vi "Single Station Execution.vi"() -> ()   [LabVIEW 2015, in "Single Station Execution.lvlib"]
uses:
  Single Station Execution.lvlib
  Types/Log.SelectedChannels.ctl
  Types/Main.StateVariables.ctl
  Types/INI.Settings.ctl
  <vilib>/NI Veristand/Execution/AlarmManager/AlarmManagerAPI.ctl
  <vilib>/NI Veristand/Execution/DataLogging/IDataLogging Ref.ctl
  <vilib>/NI Veristand/Execution/DataLogging/DataLoggingSpecification Ref.ctl
  Types/Execute.UserEventRefs.ctl
  <vilib>/NI Veristand/Execution/Workspace/SystemStateRegEventRef.ctl
  <vilib>/NI Veristand/Execution/Workspace/Target State Info.ctl
  <vilib>/NI Veristand/Execution/Workspace/Target State.ctl
  Types/Execution.SequenceState.ctl
  <vilib>/NI Veristand/Execution/Workspace/SystemStateEventRef.ctl
  <vilib>/NI Veristand/Execution/Workspace/WorkspaceAPI.ctl
  Types/UDPEngine.QueueCluster.ctl
  Types/UDPEngine.State.ctl
  Types/Results.Value.ctl
  NationalInstruments.VeriStand.RealTimeSequenceDefinitionApi
  <vilib>/NI/AMC/Read Termination Message.vi
  <vilib>/NI/AMC/Update Message Routing Info.vi
  <vilib>/NI/AMC/Create Multiple Messages.vi
  <vilib>/NI/AMC/Create Single Message.vi
  <vilib>/NI/AMC/Globals.vi
  <vilib>/NI/AMC/Send Message.vi
  SubVIs/Main.Constants.vi
  <vilib>/NI Veristand/Execution/Workspace/NI VeriStand - Set Single Channel Value.vi
  <vilib>/NI Veristand/Execution/Workspace/NI_VS Workspace ExecutionAPI.lvlib
  NationalInstruments.VeriStand.ClientAPI
  <vilib>/NI Veristand/Execution/DataLogging/NI_VS Data Logging API.lvlib
  <vilib>/NI/AMC/AMC.lvlib
  <vilib>/NI Veristand/Execution/AlarmManager/NI_VS AlarmManager ExecutionAPI.lvlib
panel:
  in  "ClientPort":u16
  in  "Enable Logging":bool=TRUE
  in  "Log Channels":T1=enum."Aliases"
  in  "Multihead":bool
  out "Status":string
  in  "Station.ID":string="Station_1"
  out "Station ID":string="Station 1"
  in  "NIVS.Gateway IP Address":string="localhost"
  in  "NIVS.Workspace Event":refnum<event-registration>
  in  "ToolTab":enum32{"Enable", "Disable"}(tab)
  in  "Back":bool
  in  "Next":bool
  in  "Pages":enum32{"Metadata", "Alarms", "Execution"}(tab)
  in  "Description":string
  in  "Operator Name":string
  in  "Work Order Number":string
  in  "Cyclic Frequency":dbl
  in  "Number of Cycles":u32
  out "Waveform Preview":waveform(dbl)[](graph)
  in  "Waveform Definition":path
  in  "Revert":bool
  in  "Apply":bool
  in  "Disable Alarms":bool
  out "Monitored Variable":string
  in  "Delay Time":dbl
  in  "Enable State":u16(ring) items=["Disabled", "Enabled", "Tripped", "Delayed Trip", "Indicate"]
  in  "Low":dbl
  in  "High":dbl
  in  "Alarms":i32(listbox)
  in  "Base File Name":string="Log" caption="Base File Name (timestamp included automatically)"
  out "Table":i32(listbox)
  in  "View":enum16{"Graph", "Table"}(ring)
  out "Chart":waveform(dbl)[](graph)
  out "Profile":string
  in  "Run":bool
  in  "Pause":bool
  in  "Abort":bool
  in  "Start Iteration":u32 min=1 max=50
  in  "Start Step":u32 min=1 max=1
  out "Current Iteration":u32 min=1 max=2
  out "Current Step":u32 min=1 max=5
  out "Total Iterations":u32 min=1 max=2
  in  "Skip":bool
  out "Duration":dbl min=1.0 max=3.0
  in  "Open Alarm":bool
  in  "Open Log Directory":bool
  in  "Open Report":bool
  out "Alarm Log Path":path
  in  "Ack":bool
  out "Result":string
  out "Restart Path":path
  out "Report Path":path
  out "Log Directory":path
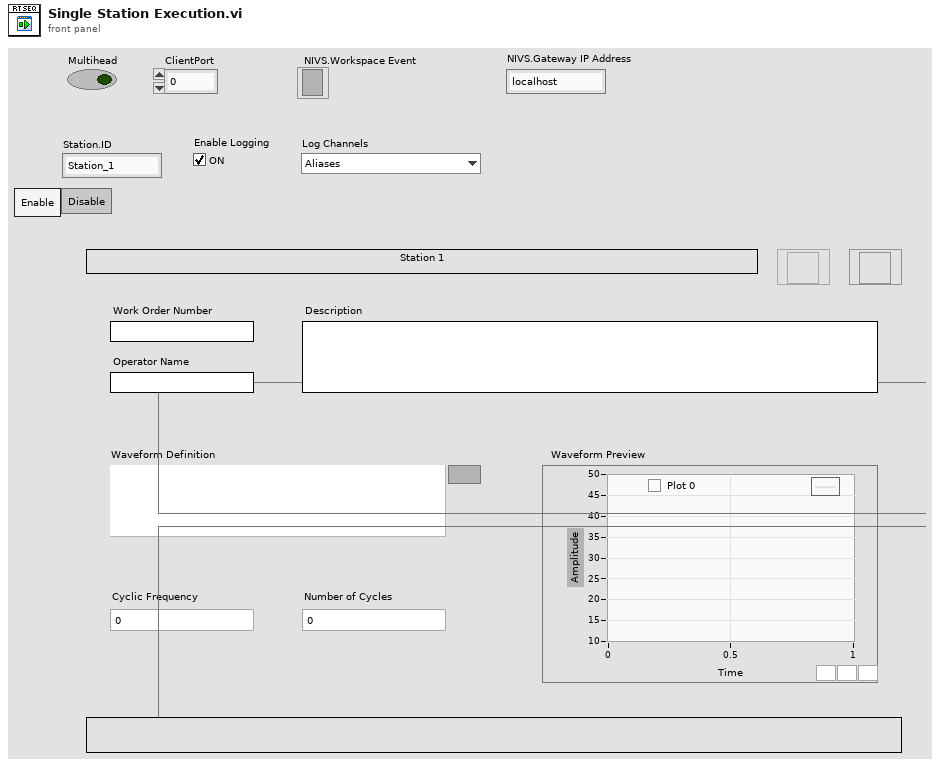
[diagram p1: front panel]
types:
  T1 = typedef "Single Station Execution.lvlib/Log.SelectedChannels.ctl" = enum16{"Channels (No System Channel)", "Aliases", "All"}
  T2 = typedef "Single Station Execution.lvlib/UDPEngine.QueueCluster.ctl" = cluster{"Action":T3, "Channels":string[]}
  T3 = typedef "Single Station Execution.lvlib/UDPEngine.State.ctl" = enum8{"Idle", "Start Acq", "Run", "Stop Acq", "Exit"}
  T4 = typedef "Single Station Execution.lvlib/Execution.SequenceState.ctl" = enum16{"Idle", "Initializing", "Running", "Paused", "Finalizing", "Complete"}
  T5 = typedef "Single Station Execution.lvlib/Main.StateVariables.ctl" = cluster{"Events.State":refnum<user-event>, "Events.Test Result":refnum<user-event>, "Events.Progress":refnum<user-event>, "INI.Settings":T6, "NIVS.AlarmManager":T7, "NIVS.BaseLogPath":path, "NIVS.DataLogManagerRef":T8, "NIVS.DataLogSpecRef":T9, "NIVS.Deployed":bool, "NIVS.Events":T10, "NIVS.GatewayIPAddress":string, "NIVS.DataLogGUID":string, "NIVS.ProfileCallback":refnum<k27>, "NIVS.ProfileRef":refnum<k24>, "NIVS.SequenceState":T4, "NIVS.SystemDefinitionFile":path, "NIVS.SystemStateRefs":T12, "NIVS.WorkspaceManager":T13, "NIVS.EventLogGUID":string, "NIVS.EventLogManagerRef":T8, "NIVS.EventLogSpecRef":T9, "NIVS.BaseToolPath":path, "Restart.Path":path, "Sequence.#ofColumns":i32, "Sequence.Iterations":u32, "Sequence.Channels":string[], "Sequence.ValidConfig?":bool, "Station.ID":string, "UDP.Queue":refnum<queue>, "UI.Abort":refnum<vi>, "UI.Alarms":refnum<vi>, "UI.Apply":refnum<vi>, "UI.Back":refnum<vi>, "UI.BaseFileName":refnum<vi>, "UI.CurrentIteration":refnum<vi>, "UI.CurrentStep":refnum<vi>, "UI.CyclicFrequency":refnum<vi>, "UI.Description":refnum<vi>, "UI.DelayTime":refnum<vi>, "UI.DisableAlarms":refnum<vi>, "UI.Duration":refnum<vi>, "UI.EnableLogging":refnum<vi>, "UI.EnableState":refnum<vi>, "UI.High":refnum<vi>, "UI.LogChannels":refnum<vi>, "UI.Low":refnum<vi>, "UI.MonitoredVariable":refnum<vi>, "UI.Next":refnum<vi>, "UI.NumberOfCycles":refnum<vi>, "UI.OperatorName":refnum<vi>, "UI.Pause":refnum<vi>, "UI.Profile":refnum<vi>, "UI.Revert":refnum<vi>, "UI.Skip":refnum<vi>, "UI.Start":refnum<vi>, "UI.StartIteration":refnum<vi>, "UI.StartStep":refnum<vi>, "UI.TabControl":refnum<vi>, "UI.TotalIterations":refnum<vi>, "UI.WaveformDefinition":refnum<vi>, "UI.WaveformPreview":refnum<vi>, "UI.WorkOrderNumber":refnum<vi>, "UI.Chart":refnum<vi>, "UI.Status":refnum<vi>, "UI.DataView":refnum<vi>, "UI.Table":refnum<vi>, "UI.Multihead":refnum<vi>, "UI.ToolTab":refnum<vi>, "UI.Result":refnum<vi>, "UI.Log Path":refnum<vi>, "UI.ReportPath":refnum<vi>, "UI.RestartPath":refnum<vi>, "UI.AlarmLog":refnum<vi>}
  T6 = typedef "Single Station Execution.lvlib/INI.Settings.ctl" = cluster{"Build Location":path, "LoggingLocation":path, "Sequence.AbortChannel":string, "Sequence.IterationInfoChannel":string, "Sequence.DurationChannel":string, "Sequence.StepInfoChannel":string, "Sequence.SkipChannel":string, "PlotChannels":string[], "Sequence.InitializeScript":path, "Sequence.CleanupScript":path, "Log.DefaultRate":dbl}
  T7 = typedef "NI_VS AlarmManager ExecutionAPI.lvlib/AlarmManagerAPI.ctl" = refnum<k24>
  T8 = typedef "NI_VS Data Logging API.lvlib/IDataLogging Ref.ctl" = refnum<k24>
  T9 = typedef "NI_VS Data Logging API.lvlib/DataLoggingSpecification Ref.ctl" = refnum<k24>
  T10 = typedef "Single Station Execution.lvlib/Execute.UserEventRefs.ctl" = cluster{"SequenceEvent":refnum<event-registration>, "SystemChangeEvent":T11, "WorkspaceEvent":refnum<event-registration>}
  T11 = typedef "NI_VS Workspace ExecutionAPI.lvlib/SystemStateRegEventRef.ctl" = refnum<event-registration>
  T12 = typedef "NI_VS Workspace ExecutionAPI.lvlib/SystemStateEventRef.ctl" = cluster{"CustDatRef":refnum<user-event>, "EvtRef":refnum<k27>, "Target State User Event":refnum<user-event>}
  T13 = typedef "NI_VS Workspace ExecutionAPI.lvlib/WorkspaceAPI.ctl" = refnum<k24>
  T14 = typedef "AMC.lvlib/Message Queue.ctl" = refnum<queue>
  T15 = enum8{"Enabled", "Disabled", "Disabled and Grayed Out"}
  T16 = typedef "Single Station Execution.lvlib/Results.Value.ctl" = enum8{"Passed", "Failed", "Aborted"}
  T17 = typedef "AMC.lvlib/Message.ctl" = cluster{"name":string, "value":string, "attributes":T18, "receiver host":string, "receiver process":string, "source host":string, "source process":string, "priority message":bool, "acknowledge message":bool}
  T18 = typedef "Tools_KeyedArray.lvlib/KeyedArray.ctl" = cluster{"keys":string[], "values":string[]}
  T19 = typedef "NI_VS Workspace ExecutionAPI.lvlib/SystemState.ctl" = u8
  T20 = typedef "Single Station Execution.lvlib/Stimulus.Status.ctl" = cluster{"Restart":bool, "NIVS.SequenceState":T4, "Alarmed?":bool, "Disable?":bool}
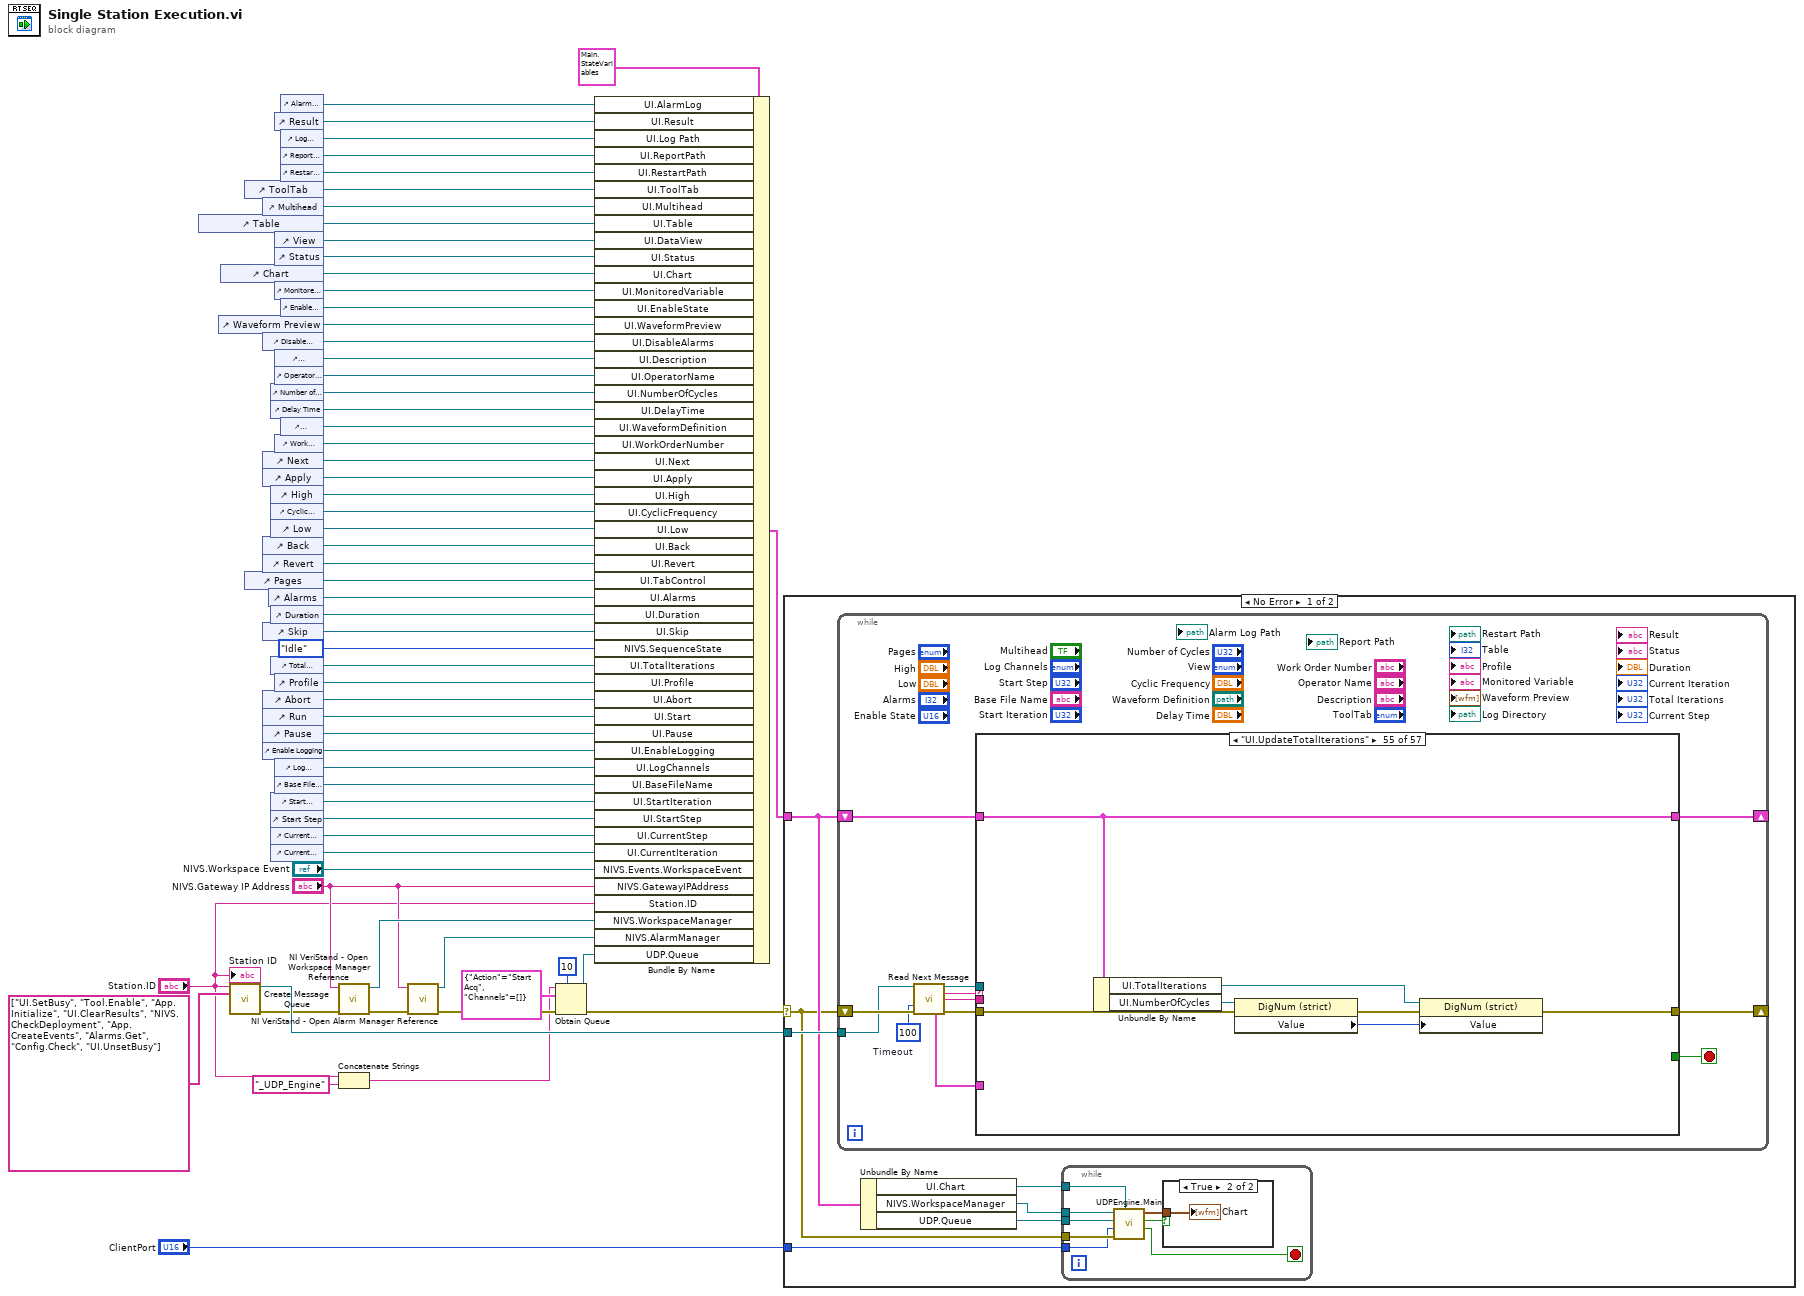
[diagram p0: block diagram]
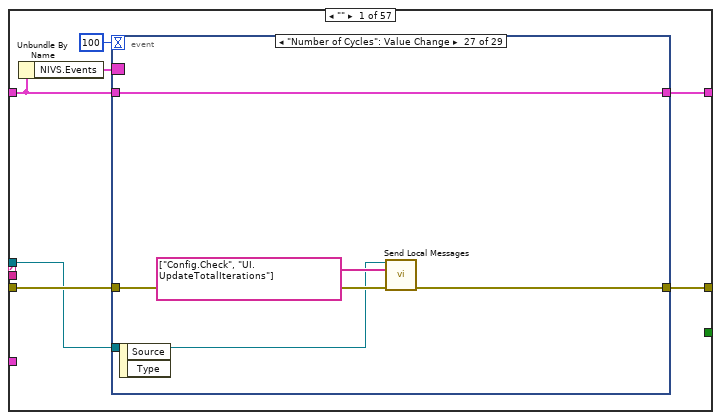
[diagram p3: hidden frame]
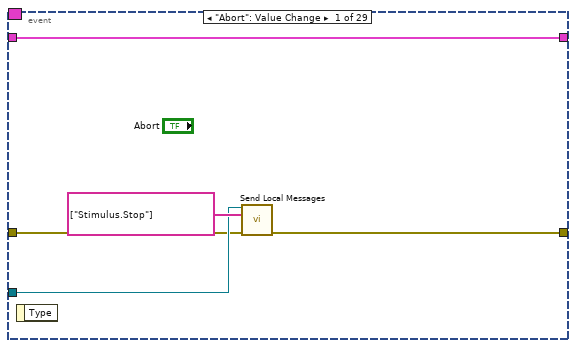
[diagram p4: hidden frame]
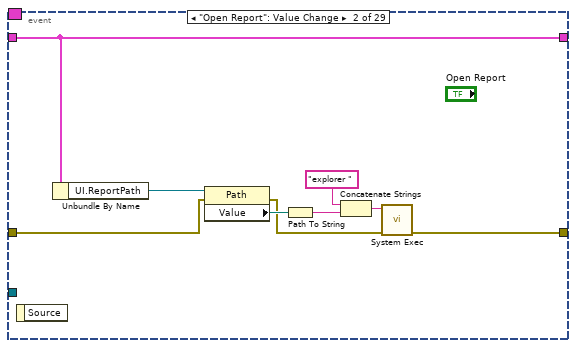
[diagram p5: hidden frame]
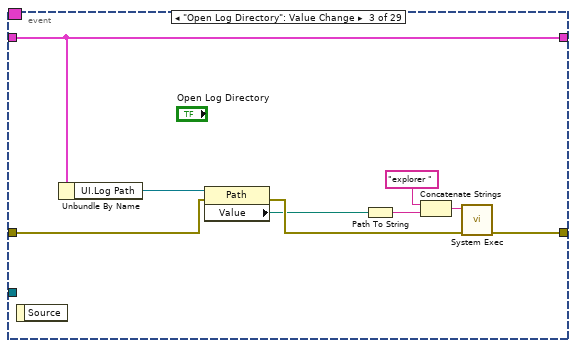
[diagram p6: hidden frame]
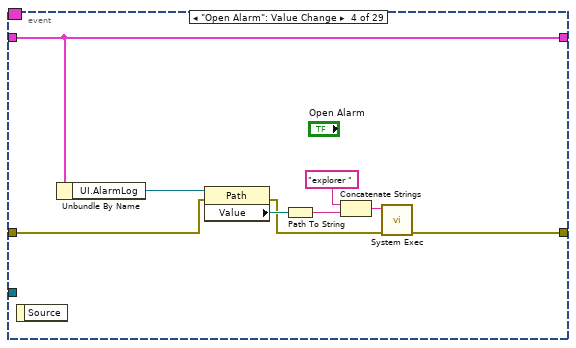
[diagram p7: hidden frame]
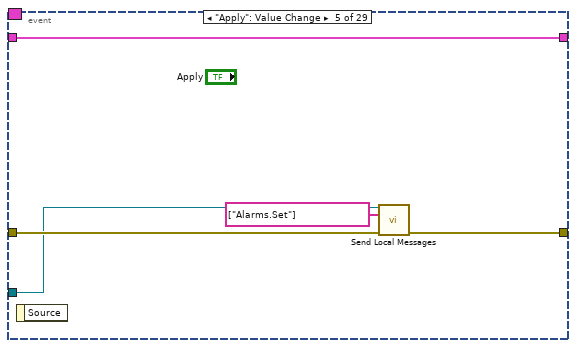
[diagram p8: hidden frame]
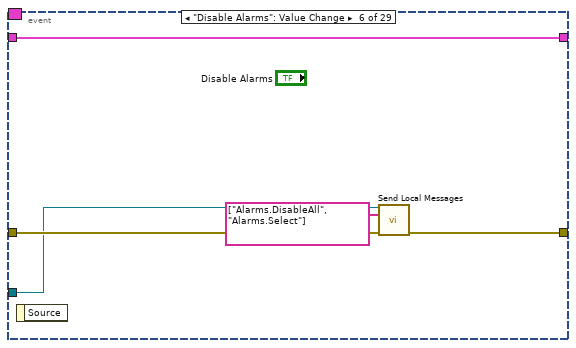
[diagram p9: hidden frame]
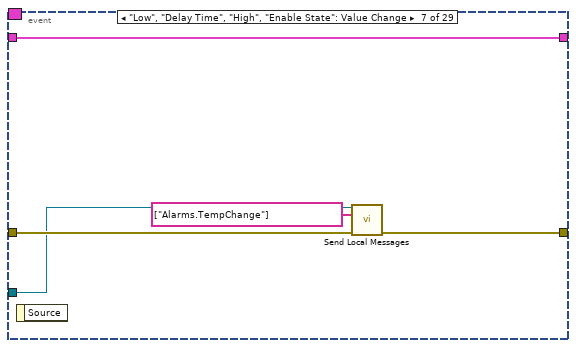
[diagram p10: hidden frame]
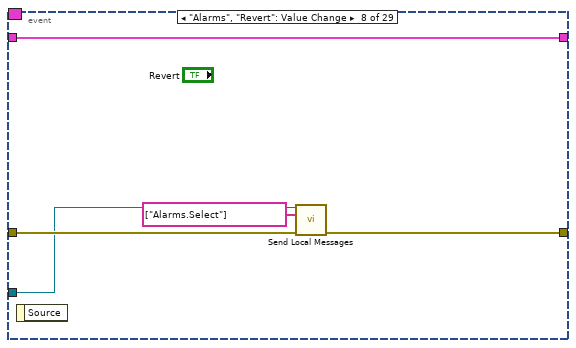
[diagram p11: hidden frame]
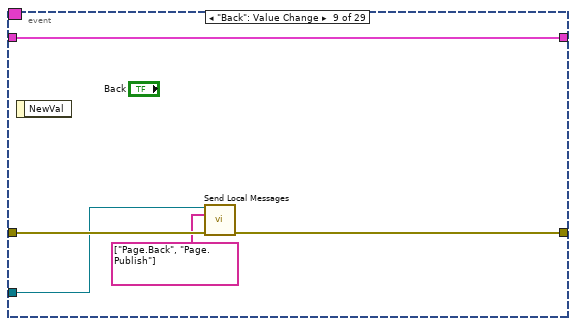
[diagram p12: hidden frame]
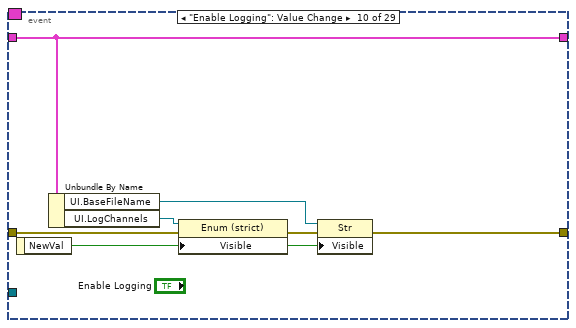
[diagram p13: hidden frame]
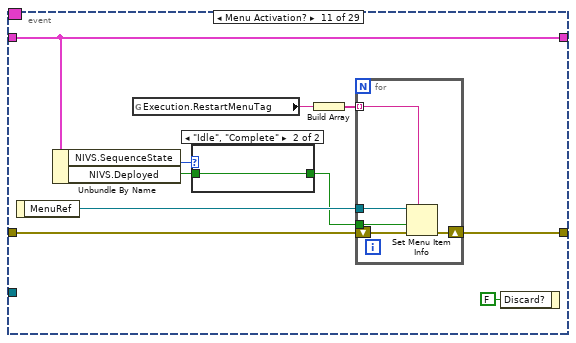
[diagram p14: hidden frame]
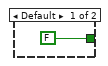
[diagram p15: hidden frame]
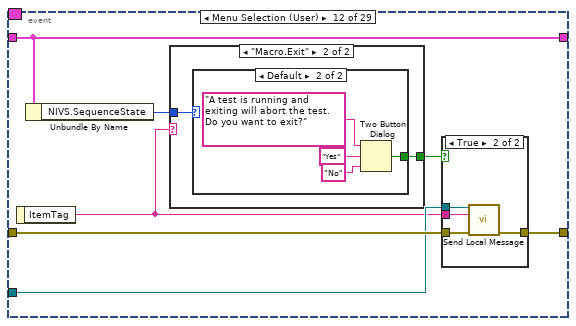
[diagram p16: hidden frame]
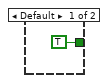
[diagram p18: hidden frame]
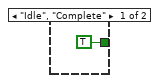
[diagram p19: hidden frame]
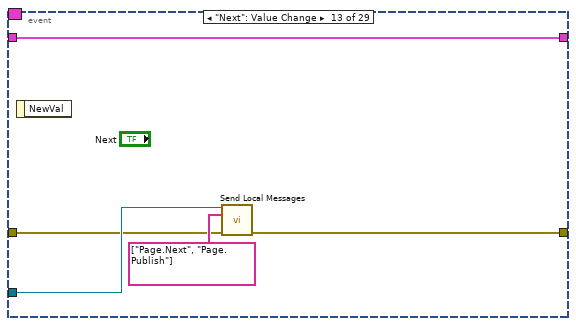
[diagram p20: hidden frame]
diagram:
  n1 = control-ref of="Table"() -> (w12:refnum<vi>)
  n2 = control-ref of="Waveform Preview"() -> (w22:refnum<vi>)
  n3 = control-ref of="Chart"() -> (w14:refnum<vi>)
  n4 = call <vilib>:"Create Message Queue.vi"("message queue name"="Station.ID", "initial message names"=string[] ["UI.SetBusy", "Tool.Enable", "App.Initialize", "UI.ClearResults", "NIVS.CheckDeployment", "App.CreateEvents", "Alarms.Get", "Config.Check", "UI.UnsetBusy"]) -> ("message queue out"=w45:T14, "error out"=w27:errorcluster)  [unwired: 12 in]
  n5 = control-ref of="ToolTab"() -> (w7:refnum<vi>)
  n6 = control-ref of="Pages"() -> (w23:refnum<vi>)
  n7 = control-ref of="Multihead"() -> (w8:refnum<vi>)
  n8 = control-ref of="Disable Alarms"() -> (w30:refnum<vi>)
  n9 = control-ref of="Next"() -> (w36:refnum<vi>)
  n10 = control-ref of="Apply"() -> (w37:refnum<vi>)
  n11 = control-ref of="Back"() -> (w41:refnum<vi>)
  n12 = control-ref of="Revert"() -> (w42:refnum<vi>)
  n13 = control-ref of="Skip"() -> (w47:refnum<vi>)
  n14 = control-ref of="Abort"() -> (w64:refnum<vi>)
  n15 = control-ref of="Run"() -> (w63:refnum<vi>)
  n16 = control-ref of="Pause"() -> (w62:refnum<vi>)
  n17 = control-ref of="Enable Logging"() -> (w61:refnum<vi>)
  n18 = control-ref of="Alarms"() -> (w43:refnum<vi>)
  n19 = control-ref of="Number of Cycles"() -> (w21:refnum<vi>)
  n20 = control-ref of="Delay Time"() -> (w33:refnum<vi>)
  n21 = control-ref of="High"() -> (w38:refnum<vi>)
  n22 = control-ref of="Cyclic Frequency"() -> (w39:refnum<vi>)
  n23 = control-ref of="Low"() -> (w40:refnum<vi>)
  n24 = control-ref of="Duration"() -> (w46:refnum<vi>)
  n25 = control-ref of="Total Iterations"() -> (w50:refnum<vi>)
  n26 = control-ref of="Start Iteration"() -> (w59:refnum<vi>)
  n27 = control-ref of="Start Step"() -> (w58:refnum<vi>)
  n28 = control-ref of="Current Step"() -> (w52:refnum<vi>)
  n29 = control-ref of="Current Iteration"() -> (w51:refnum<vi>)
  n30 = control-ref of="Result"() -> (w3:refnum<vi>)
  n31 = control-ref of="View"() -> (w13:refnum<vi>)
  n32 = control-ref of="Status"() -> (w20:refnum<vi>)
  n33 = control-ref of="Monitored Variable"() -> (w24:refnum<vi>)
  n34 = control-ref of="Description"() -> (w31:refnum<vi>)
  n35 = control-ref of="Operator Name"() -> (w32:refnum<vi>)
  n36 = control-ref of="Work Order Number"() -> (w35:refnum<vi>)
  n37 = control-ref of="Profile"() -> (w56:refnum<vi>)
  n38 = control-ref of="Log Channels"() -> (w60:refnum<vi>)
  n39 = control-ref of="Base File Name"() -> (w49:refnum<vi>)
  n40 = control-ref of="Alarm Log Path"() -> (w2:refnum<vi>)
  n41 = control-ref of="Log Directory"() -> (w4:refnum<vi>)
  n42 = control-ref of="Report Path"() -> (w5:refnum<vi>)
  n43 = control-ref of="Restart Path"() -> (w6:refnum<vi>)
  n44 = control-ref of="Enable State"() -> (w29:refnum<vi>)
  n45 = control-ref of="Waveform Definition"() -> (w34:refnum<vi>)
  n46 = call <vilib>:"NI VeriStand - Open Workspace Manager Reference.vi"("error in (no error)"=w27, "Gateway IP Address (\"\": localhost)"="NIVS.Gateway IP Address") -> ("error out"=w26:errorcluster, "WorkspaceManager"=w53:T13)  [unwired: 8 in]
  n47 = Concatenate Strings("Station.ID", "_UDP_Engine" ("string")) -> (w9:string)
  n48 = call <vilib>:"NI VeriStand - Open Alarm Manager Reference.vi"("error in (no error)"=w26, "Gateway IP Address (\"\": localhost)"="NIVS.Gateway IP Address") -> ("error out"=w17:errorcluster, "AlarmManager"=w28:T7)  [unwired: 8 in]
  n49 = Obtain Queue(max queue size (-1, unlimited)=10, name (unnamed)=w9, element data type=T2 {"Action"=enum."Start Acq", "Channels"=[]}, error in (no error)=w17) -> (queue out=w15:refnum<queue>, error out=w16:errorcluster)  [unwired: 1 in, 1 out]
  n50 = Bundle By Name(cluster=T5 {"Events.State"=refnum, "Events.Test Result"=refnum, "Events.Progress"=refnum, "INI.Settings"={"Build Location"=path "", "LoggingLocation"=path "", "Sequence.AbortChannel"="", "Sequence.IterationInfoChannel"="", "Sequence.DurationChannel"="", "Sequence.StepInfoChannel"="", "Sequence.SkipChannel"="", "PlotChannels"=[], "Sequence.InitializeScript"=path "C:/Simple Sequence Editor/SequenceRepo", "Sequence.CleanupScript"=path "", "Log.DefaultRate"=0.0}, "NIVS.AlarmManager"=refnum, "NIVS.BaseLogPath"=path "", "NIVS.DataLogManagerRef"=refnum, "NIVS.DataLogSpecRef"=refnum, "NIVS.Deployed"=FALSE, "NIVS.Events"={"SequenceEvent"=refnum, "SystemChangeEvent"=refnum, "WorkspaceEvent"=refnum}, "NIVS.GatewayIPAddress"="", "NIVS.DataLogGUID"="", "NIVS.ProfileCallback"=refnum, "NIVS.ProfileRef"=refnum, "NIVS.SequenceState"=enum."Idle", "NIVS.SystemDefinitionFile"=path "", "NIVS.SystemStateRefs"={"CustDatRef"=refnum, "EvtRef"=refnum, "Target State User Event"=refnum}, "NIVS.WorkspaceManager"=refnum, "NIVS.EventLogGUID"="", "NIVS.EventLogManagerRef"=refnum, "NIVS.EventLogSpecRef"=refnum, "NIVS.BaseToolPath"=path "", "Restart.Path"=path "", "Sequence.#ofColumns"=0, "Sequence.Iterations"=0, "Sequence.Channels"=[], "Sequence.ValidConfig?"=FALSE, "Station.ID"="", "UDP.Queue"=refnum, "UI.Abort"=refnum, "UI.Alarms"=refnum, "UI.Apply"=refnum, "UI.Back"=refnum, "UI.BaseFileName"=refnum, "UI.CurrentIteration"=refnum, "UI.CurrentStep"=refnum, "UI.CyclicFrequency"=refnum, "UI.Description"=refnum, "UI.DelayTime"=refnum, "UI.DisableAlarms"=refnum, "UI.Duration"=refnum, "UI.EnableLogging"=refnum, "UI.EnableState"=refnum, "UI.High"=refnum, "UI.LogChannels"=refnum, "UI.Low"=refnum, "UI.MonitoredVariable"=refnum, "UI.Next"=refnum, "UI.NumberOfCycles"=refnum, "UI.OperatorName"=refnum, "UI.Pause"=refnum, "UI.Profile"=refnum, "UI.Revert"=refnum, "UI.Skip"=refnum, "UI.Start"=refnum, "UI.StartIteration"=refnum, "UI.StartStep"=refnum, "UI.TabControl"=refnum, "UI.TotalIterations"=refnum, "UI.WaveformDefinition"=refnum, "UI.WaveformPreview"=refnum, "UI.WorkOrderNumber"=refnum, "UI.Chart"=refnum, "UI.Status"=refnum, "UI.DataView"=refnum, "UI.Table"=refnum, "UI.Multihead"=refnum, "UI.ToolTab"=refnum, "UI.Result"=refnum, "UI.Log Path"=refnum, "UI.ReportPath"=refnum, "UI.RestartPath"=refnum, "UI.AlarmLog"=refnum} ("Cluster"), "UI.AlarmLog"=w2, "UI.Result"=w3, "UI.Log Path"=w4, "UI.ReportPath"=w5, "UI.RestartPath"=w6, "UI.ToolTab"=w7, "UI.Multihead"=w8, "UI.Table"=w12, "UI.DataView"=w13, "UI.Status"=w20, "UI.Chart"=w14, "UI.MonitoredVariable"=w24, "UI.EnableState"=w29, "UI.WaveformPreview"=w22, "UI.DisableAlarms"=w30, "UI.Description"=w31, "UI.OperatorName"=w32, "UI.NumberOfCycles"=w21, "UI.DelayTime"=w33, "UI.WaveformDefinition"=w34, "UI.WorkOrderNumber"=w35, "UI.Next"=w36, "UI.Apply"=w37, "UI.High"=w38, "UI.CyclicFrequency"=w39, "UI.Low"=w40, "UI.Back"=w41, "UI.Revert"=w42, "UI.TabControl"=w23, "UI.Alarms"=w43, "UI.Duration"=w46, "UI.Skip"=w47, "NIVS.SequenceState"=Execution.SequenceState."Idle", "UI.TotalIterations"=w50, "UI.Profile"=w56, "UI.Abort"=w64, "UI.Start"=w63, "UI.Pause"=w62, "UI.EnableLogging"=w61, "UI.LogChannels"=w60, "UI.BaseFileName"=w49, "UI.StartIteration"=w59, "UI.StartStep"=w58, "UI.CurrentStep"=w52, "UI.CurrentIteration"=w51, "NIVS.Events.WorkspaceEvent"="NIVS.Workspace Event", "NIVS.GatewayIPAddress"="NIVS.Gateway IP Address", "Station.ID"="Station.ID", "NIVS.WorkspaceManager"=w53, "NIVS.AlarmManager"=w28, "UDP.Queue"=w15) -> (w57:T5)
  n51 = case shown="No Error" w16 {
    selector: w16 -> [w66 _]
    tunnel: w57 -> [w70 _]
    tunnel: w45 -> [w71 _]
    tunnel: "ClientPort" -> [w65 _]
    frame No Error {
      n52 = while {
        shift-right: [w91] -> _
        shift-left: w70 -> [w92]
        shift-right: [w81] -> _
        shift-left: w66 -> [w90]
        tunnel: w71 -> [w88]
        stop <- w89 stop-if-true
        w87 = 100  # Timeout
        n53 = call <vilib>:"Read Next Message.vi"("message queue in"=w88, "timeout (1 ms)"=w87, "error in"=w90) -> ("message queue out"=w85:T14, "message name"=w84:string, "message value"=w83:string, "message"=w82:T17, "error out"=w86:errorcluster)  [unwired: 5 in, 3 out]
        n54 = case shown="\"UI.UpdateTotalIterations\"" w84 {
          selector: w84 -> [_ _ _ _ _ _ _ _ _ _ _ _ _ _ _ _ _ _ _ _ _ _ _ _ _ _ _ _ _ _ _ _ _ _ _ _ _ w707 _ _ _ _ _ _ _ w775 _ _ _ w790 _ _ _ _ _ _ _]
          tunnel: w92 -> [w95 w361 w373 w378 w383 w386 w393 w398 w401 w405 w416 w429 w440 w449 w459 w465 w492 w505 w525 w544 w569 w574 w588 w593 w598 w606 w609 w630 w661 w665 w670 w675 w676 w682 w687 w693 w699 w709 w715 w722 w730 w741 w747 w768 w774 w779 w780 w783 w786 w793 w807 w817 w827 w855 w866 w874 w876]
          tunnel: [w99 w361 w373 w378 w383 w386 w393 w398 w401 w404 w418 w429 w440 w452 w459 w472 w491 w505 w525 w544 w569 w574 w588 w593 w598 w605 w609 w630 w661 w665 w670 w675 w676 w680 w686 w693 w698 w709 w714 w722 w731 w740 w747 w768 w774 w779 w780 w783 w786 w793 w807 w817 w827 w855 w866 w874 w876] -> w91
          tunnel: [w96 w358 w370 w375 w379 w387 w389 w396 w402 w412 w419 w427 w441 w453 w456 w469 w498 w507 w529 w549 w567 w572 w585 w589 w594 w602 w611 w629 w647 w662 w667 w672 w677 w684 w688 w689 w700 w702 w716 w718 w737 w739 w748 w769 w772 w776 w781 w784 w787 w789 w798 w816 w823 w848 w860 w869 w875] -> w81
          tunnel: w86 -> [w97 w359 w371 w376 w384 w385 w392 w397 w403 w412 w417 w426 w442 w454 w457 w470 w500 w510 w532 w548 w568 w573 w586 w590 w595 w604 w610 w628 w647 w663 w668 w673 w678 w685 w688 w690 w701 w704 w717 w719 w738 w742 w749 w769 w773 w776 w782 w785 w788 w789 w797 w815 w820 w850 w861 w870 w875]
          tunnel: [_ _ _ _ _ _ _ _ _ _ _ _ TRUE _ _ _ _ _ _ _ _ _ _ _ _ _ _ _ _ _ _ _ _ _ _ _ _ _ _ _ _ _ _ _ _ _ _ _ _ _ _ _ _ _ _ _ _] -> w89
          tunnel: w85 -> [w93 _ _ _ w381 _ w388 _ _ _ _ _ w443 _ w458 w460 w497 w504 _ w545 _ w571 w584 w591 w596 w601 _ _ _ _ _ _ _ _ _ _ _ _ _ _ _ _ _ _ _ _ _ _ _ _ _ _ _ _ _ _ _]
          tunnel: w83 -> [_ _ _ _ _ _ _ _ _ _ _ _ _ _ _ _ _ _ _ _ _ _ _ _ _ _ _ _ _ w664 _ _ _ _ _ _ _ _ _ _ _ _ _ _ _ _ _ _ _ _ _ _ w821 _ _ _ _]
          tunnel: w82 -> [_ _ _ _ _ _ _ _ _ _ _ _ _ _ _ _ _ _ _ _ _ _ _ _ _ _ _ _ _ _ _ _ _ _ _ _ _ w713 _ _ _ _ _ _ _ _ _ _ _ _ _ _ _ _ _ _ _]
          frame "" {
            n55 = Unbundle By Name(w95) -> ("NIVS.Events"=w94:T10)
            n56 = event shown="[26] \"Number of Cycles\": Value Change" {
              selector: w94 -> [_ _ _ _ _ _ _ _ _ _ _ _ _ _ _ _ _ _ _ _ _ _ _ _ _ _ _ _ _]
              dyn-events: _ -> [_ _ _ _ _ _ _ _ _ _ _ _ _ _ _ _ _ _ _ _ _ _ _ _ _ _ _ _ _]
              timeout: 100 -> [_ _ _ _ _ _ _ _ _ _ _ _ _ _ _ _ _ _ _ _ _ _ _ _ _ _ _ _ _]
              tunnel: [w104 w113 w122 w131 w136 w141 w146 w151 w156 w163 w173 w181 w205 w211 w217 w225 w244 w245 w263 w269 w279 w302 w306 w313 w318 w323 w328 w337 w345] -> w99
              tunnel: w95 -> [w104 w113 w122 w131 w136 w141 w146 w151 w156 w163 w173 w181 w205 w211 w217 w225 w244 w256 w263 w270 w279 w302 w306 w313 w318 w323 w328 w337 w345]
              tunnel: [w100 w105 w115 w123 w133 w138 w144 w149 w154 w157 w169 w186 w203 w208 w215 w218 w243 w250 w261 w264 w275 w297 w307 w311 w316 w320 w325 w332 w342] -> w96
              tunnel: w97 -> [w101 w111 w120 w129 w134 w139 w145 w150 w155 w161 w170 w187 w201 w209 w216 w222 w243 w246 w262 w268 w276 w298 w308 w312 w317 w321 w326 w333 w343]
              tunnel: w93 -> [w102 _ _ _ w132 w137 w143 w148 w153 _ _ w185 w202 w207 w214 w220 _ w248 w260 w267 _ w299 _ w309 w314 w319 w324 _ w341]
              event "Abort": Value Change {
                n57 = event-data() -> ()  [unwired: 1 in, 1 out]
                n58 = call <vilib>:"Send Local Messages.vi"("message queue in"=w102, "message names"=string[] ["Stimulus.Stop"] ("array"), "error in"=w101) -> ("error out"=w100:errorcluster)  [unwired: 10 in, 2 out]
              }
              event "Open Report": Value Change {
                n59 = event-data() -> ()  [unwired: 1 in, 1 out]
                n60 = Unbundle By Name(w113) -> ("UI.ReportPath"=w112:refnum<vi>)
                n61 = property class="Path"(reference=w112, error in=w111) -> (error out=w106:errorcluster, "Value"=w107:path)  [unwired: 1 out]
                n62 = Path To String(path=w107) -> (string=w110:string)
                n63 = Concatenate Strings("explorer " ("string"), w110) -> (w108:string)
                n64 = call <vilib>:"System Exec.vi"("error in (no error)"=w106, "command line"=w108) -> ("error out"=w105:errorcluster)  [unwired: 6 in, 3 out]
              }
              event "Open Log Directory": Value Change {
                n65 = event-data() -> ()  [unwired: 1 in, 1 out]
                n66 = Unbundle By Name(w122) -> ("UI.Log Path"=w121:refnum<vi>)
                n67 = property class="Path"(reference=w121, error in=w120) -> (error out=w116:errorcluster, "Value"=w114:path)  [unwired: 1 out]
                n68 = Path To String(path=w114) -> (string=w119:string)
                n69 = Concatenate Strings("explorer " ("string"), w119) -> (w117:string)
                n70 = call <vilib>:"System Exec.vi"("error in (no error)"=w116, "command line"=w117) -> ("error out"=w115:errorcluster)  [unwired: 6 in, 3 out]
              }
              event "Open Alarm": Value Change {
                n71 = event-data() -> ()  [unwired: 1 in, 1 out]
                n72 = Unbundle By Name(w131) -> ("UI.AlarmLog"=w130:refnum<vi>)
                n73 = property class="Path"(reference=w130, error in=w129) -> (error out=w124:errorcluster, "Value"=w125:path)  [unwired: 1 out]
                n74 = Path To String(path=w125) -> (string=w128:string)
                n75 = Concatenate Strings("explorer " ("string"), w128) -> (w126:string)
                n76 = call <vilib>:"System Exec.vi"("error in (no error)"=w124, "command line"=w126) -> ("error out"=w123:errorcluster)  [unwired: 6 in, 3 out]
              }
              event "Apply": Value Change {
                n77 = event-data() -> ()  [unwired: 1 in, 1 out]
                n78 = call <vilib>:"Send Local Messages.vi"("message queue in"=w132, "message names"=string[] ["Alarms.Set"], "error in"=w134) -> ("error out"=w133:errorcluster)  [unwired: 10 in, 2 out]
              }
              event "Disable Alarms": Value Change {
                n79 = event-data() -> ()  [unwired: 1 in, 1 out]
                n80 = call <vilib>:"Send Local Messages.vi"("message queue in"=w137, "message names"=string[] ["Alarms.DisableAll", "Alarms.Select"], "error in"=w139) -> ("error out"=w138:errorcluster)  [unwired: 10 in, 2 out]
              }
              event "Low", "Delay Time", "High", "Enable State": Value Change {
                n81 = event-data() -> ()  [unwired: 1 in, 1 out]
                n82 = call <vilib>:"Send Local Messages.vi"("message queue in"=w143, "message names"=string[] ["Alarms.TempChange"], "error in"=w145) -> ("error out"=w144:errorcluster)  [unwired: 10 in, 2 out]
              }
              event "Alarms", "Revert": Value Change {
                n83 = event-data() -> ()  [unwired: 1 in, 1 out]
                n84 = call <vilib>:"Send Local Messages.vi"("message queue in"=w148, "message names"=string[] ["Alarms.Select"], "error in"=w150) -> ("error out"=w149:errorcluster)  [unwired: 10 in, 2 out]
              }
              event "Back": Value Change {
                n85 = event-data() -> ()  [unwired: 1 in, 1 out]
                n86 = call <vilib>:"Send Local Messages.vi"("message queue in"=w153, "message names"=string[] ["Page.Back", "Page.Publish"], "error in"=w155) -> ("error out"=w154:errorcluster)  [unwired: 10 in, 2 out]
              }
              event "Enable Logging": Value Change {
                n87 = event-data() -> ("NewVal"=w158:bool)  [unwired: 1 in]
                n88 = Unbundle By Name(w163) -> ("UI.BaseFileName"=w159:refnum<vi>, "UI.LogChannels"=w162:refnum<vi>)
                n89 = property class="Enum (strict)"(reference=w162, error in=w161, "Visible"=w158) -> (error out=w160:errorcluster)  [unwired: 1 out]
                n90 = property class="Str"(reference=w159, error in=w160, "Visible"=w158) -> (error out=w157:errorcluster)  [unwired: 1 out]
              }
              event Menu Activation? {
                n91 = event-data() -> ("MenuRef"=w171:refnum<k9>)  [unwired: 1 in]
                n92 = Unbundle By Name(w173) -> ("NIVS.SequenceState"=w172:T4, "NIVS.Deployed"=w164:bool)
                n93 = global read "Main.Constants.vi" "Execution.RestartMenuTag"() -> (w167:string)
                n94 = case shown="\"Idle\", \"Complete\"" w172 {
                  tunnel: [FALSE w180] -> w168
                  tunnel: w164 -> [_ w180]
                  frame Default {
                  }
                  frame "Idle", "Complete" {
                  }
                }
                n95 = Build Array(w167) -> (w166:string[])
                n96 = for {
                  tunnel: w171 -> [w178]
                  shift-right: [w176] -> w169
                  shift-left: w170 -> [w177]
                  tunnel: w168 -> [w175]
                  tunnel: w166 -> [w174] mode=indexing
                  n97 = Set Menu Item Info(7:w174, 8:w177, 9:w175, 11:w178) -> (0:w176:errorcluster)  [unwired: 3 in, 1 out]
                }
                n98 = event-data("Discard?"=FALSE) -> ()  [unwired: 1 in, 1 out]
              }
              event Menu Selection (User) {
                n99 = event-data() -> ("ItemTag"=w184:string)  [unwired: 1 in]
                n100 = Unbundle By Name(w181) -> ("NIVS.SequenceState"=w182:T4)
                n101 = case shown="\"Macro.Exit\"" w184 {
                  tunnel: [TRUE ("T button?") w195] -> w183
                  tunnel: w182 -> [_ w194]
                  frame Default {
                  }
                  frame "Macro.Exit" {
                    n102 = case shown="Default" w194 {
                      tunnel: [TRUE ("T button?") w197] -> w195
                      frame "Idle", "Complete" {
                      }
                      frame Default {
                        n103 = Two Button Dialog(message="A test is running and exiting will abort the test. Do you want to exit?", 1:"No" ("F button name (\"Cancel\")"), 2:"Yes" ("T button name (\"OK\")")) -> (T button?=w197:bool)
                      }
                    }
                  }
                }
                n104 = case shown="True" w183 {
                  tunnel: w187 -> [w188 w192]
                  tunnel: [w188 w191] -> w186
                  tunnel: w185 -> [_ w190]
                  tunnel: w184 -> [_ w189]
                  frame False {
                  }
                  frame True {
                    n105 = call <vilib>:"Send Local Message.vi"("message queue in"=w190, "message name"=w189, "error in"=w192) -> ("error out"=w191:errorcluster)  [unwired: 10 in, 2 out]
                  }
                }
              }
              event "Next": Value Change {
                n106 = event-data() -> ()  [unwired: 1 in, 1 out]
                n107 = call <vilib>:"Send Local Messages.vi"("message queue in"=w202, "message names"=string[] ["Page.Next", "Page.Publish"], "error in"=w201) -> ("error out"=w203:errorcluster)  [unwired: 10 in, 2 out]
              }
              event Panel Close? {
                n108 = event-data() -> ()  [unwired: 1 in, 1 out]
                n109 = Build Array("Macro.Exit") -> (w206:string[])
                n110 = call <vilib>:"Send Local Messages.vi"("message queue in"=w207, "message names"=w206, "error in"=w209) -> ("error out"=w208:errorcluster)  [unwired: 10 in, 2 out]
                n111 = event-data("Discard?"=TRUE) -> ()  [unwired: 1 in, 1 out]
              }
              event "Pause": Value Change {
                n112 = event-data() -> ()  [unwired: 1 in, 1 out]
                n113 = call <vilib>:"Send Local Messages.vi"("message queue in"=w214, "message names"=string[] ["Stimulus.Pause"] ("array"), "error in"=w216) -> ("error out"=w215:errorcluster)  [unwired: 10 in, 2 out]
              }
              event "Run": Value Change {
                n114 = event-data() -> ("CtlRef"=w223:refnum<vi>)  [unwired: 1 in]
                n115 = Unbundle By Name(w225) -> ("NIVS.SequenceState"=w224:T4)
                n116 = property class="Bool"(reference=w223, error in=w222) -> (error out=w219:errorcluster, "BoolText.Text"=w221:string)  [unwired: 1 out]
                n117 = case shown="\"Run\", Default" w221 {
                  tunnel: w224 -> [_ w233]
                  tunnel: w220 -> [w228 w232]
                  tunnel: w219 -> [w227 w231]
                  tunnel: [w226 w230] -> w218
                  frame "Restart" {
                    n118 = call <vilib>:"Send Local Messages.vi"("message queue in"=w228, "message names"=string[] ["Macro.Restart"], "error in"=w227) -> ("error out"=w226:errorcluster)  [unwired: 10 in, 2 out]
                  }
                  frame "Run", Default {
                    n119 = case shown="\"Idle\"" w233 {
                      tunnel: w232 -> [w236 _ w241]
                      tunnel: w231 -> [w235 w238 w242]
                      tunnel: [w234 w238 w240] -> w230
                      frame "Paused" {
                        n120 = call <vilib>:"Send Local Messages.vi"("message queue in"=w236, "message names"=string[] ["Stimulus.Continue"] ("array"), "error in"=w235) -> ("error out"=w234:errorcluster)  [unwired: 10 in, 2 out]
                      }
                      frame Default {
                      }
                      frame "Idle" {
                        n121 = call <vilib>:"Send Local Messages.vi"("message queue in"=w241, "message names"=string[] ["Macro.Run"] ("array"), "error in"=w242) -> ("error out"=w240:errorcluster)  [unwired: 10 in, 2 out]
                      }
                    }
                  }
                }
              }
              event User Event {
                n122 = event-data() -> ()  [unwired: 1 in, 1 out]
              }
              event User Event {
                n123 = event-data() -> ("Test Result"=w257:path)  [unwired: 1 in]
                n124 = call "Restart.HandleSequenceFinishedEvent.vi"("error in (no error)"=w246, "results path"=w257, "State Variables"=w256) -> ("error out"=w251:errorcluster, "Restart?"=w255:bool, "State Variables out"=w245:T5)  [unwired: 6 in]
                n125 = Select(t="UI.StimulusRestart", s=w255, f="UI.StimulusComplete") -> (s? t:f=w252:string)
                n126 = Build Array (concatenate)(string[] ["Stimulus.Close", "Stimulus.UnregisterCallbacks", "Acq.Stop"], w252, "Tool.Disable" ("element")) -> (w249:string[])
                n127 = call <vilib>:"Send Local Messages.vi"("message queue in"=w248, "message names"=w249, "error in"=w251) -> ("error out"=w250:errorcluster)  [unwired: 10 in, 2 out]
              }
              event "Ack": Value Change {
                n128 = event-data() -> ()  [unwired: 1 in, 1 out]
                n129 = call <vilib>:"Send Local Messages.vi"("message queue in"=w260, "message names"=string[] ["Tool.Enable", "UI.ClearResults"], "error in"=w262) -> ("error out"=w261:errorcluster)  [unwired: 10 in, 2 out]
              }
              event User Event {
                n130 = event-data() -> ("State"=w265:i32)  [unwired: 1 in]
                n131 = Bundle By Name(cluster=w270, "NIVS.SequenceState"=w265) -> (w269:T5)
                n132 = call <vilib>:"Send Local Messages.vi"("message queue in"=w267, "message names"=string[] ["UI.UpdateState", "UI.UpdateStatus"] ("array"), "error in"=w268) -> ("error out"=w264:errorcluster)  [unwired: 10 in, 2 out]
              }
              event "Skip": Value Change {
                n133 = event-data() -> ()  [unwired: 1 in, 1 out]
                n134 = Unbundle By Name(w279) -> ("Sequence.ValidConfig?"=w273:bool, "NIVS.Deployed"=w272:bool, "NIVS.SequenceState"=w274:T4, "NIVS.WorkspaceManager"=w278:T13, "INI.Settings.Sequence.SkipChannel"=w277:string)
                n135 = Compound Arithmetic op=AND(w273, w272) -> (w271:bool)
                n136 = case shown="True" w271 {
                  tunnel: w278 -> [_ w283]
                  tunnel: w276 -> [w280 w285]
                  tunnel: [w280 w284] -> w275
                  tunnel: w277 -> [_ w282]
                  tunnel: w274 -> [_ w281]
                  frame False {
                  }
                  frame True {
                    n137 = case shown="Default" w281 {
                      tunnel: w285 -> [w286 w290]
                      tunnel: [w286 w289] -> w284
                      tunnel: w283 -> [_ w288]
                      tunnel: w282 -> [_ w287]
                      frame "Idle", "Complete" {
                      }
                      frame Default {
                        n138 = case shown="Default" w287 {
                          selector: w287 -> [_ w292]
                          tunnel: w290 -> [w291 w296]
                          tunnel: [w291 w295] -> w289
                          tunnel: w288 -> [_ w294]
                          frame "" {
                          }
                          frame Default {
                            n139 = call-poly <vilib>:"NI VeriStand - Set Channel Value.vi"("error in (no error)"=w296, "Value"=1.0, "Channel"=w292, "WorkspaceManager in"=w294) -> ("error out"=w295:errorcluster)  [unwired: 6 in, 1 out]
                          }
                        }
                      }
                    }
                  }
                }
              }
              event User Event {
                n140 = event-data() -> ()  [unwired: 1 in, 1 out]
                n141 = Unbundle By Name(w302) -> ("NIVS.SequenceState"=w301:T4)
                n142 = case shown="\"Idle\", \"Complete\"" w301 {
                  tunnel: [string[] ["Stimulus.CacheRestart", "NIVS.CheckDeployment"] w305] -> w300
                  frame Default {
                  }
                  frame "Idle", "Complete" {
                    n143 = Build Array("NIVS.CheckDeployment") -> (w305:string[])
                  }
                }
                n144 = call <vilib>:"Send Local Messages.vi"("message queue in"=w299, "message names"=w300, "error in"=w298) -> ("error out"=w297:errorcluster)  [unwired: 10 in, 2 out]
              }
              event Timeout {
                n145 = event-data() -> ()  [unwired: 1 in, 1 out]
                n146 = call "Stimulus.GetStatusInfo.vi"("error in (no error)"=w308, "Cluster"=w306) -> ("error out"=w307:errorcluster)  [unwired: 9 in]
              }
              event "Waveform Definition": Value Change {
                n147 = event-data() -> ()  [unwired: 1 in, 2 out]
                n148 = call <vilib>:"Send Local Messages.vi"("message queue in"=w309, "message names"=string[] ["Sequence.Open", "UI.UpdatePreview", "Config.Check"], "error in"=w312) -> ("error out"=w311:errorcluster)  [unwired: 10 in, 2 out]
              }
              event "Cyclic Frequency": Value Change {
                n149 = event-data() -> ()  [unwired: 1 in, 2 out]
                n150 = call <vilib>:"Send Local Messages.vi"("message queue in"=w314, "message names"=string[] ["UI.UpdatePreview", "Config.Check"], "error in"=w317) -> ("error out"=w316:errorcluster)  [unwired: 10 in, 2 out]
              }
              event "Operator Name", "Work Order Number", "Description": Value Change {
                n151 = event-data() -> ()  [unwired: 1 in, 2 out]
                n152 = call <vilib>:"Send Local Messages.vi"("message queue in"=w319, "message names"=string[] ["Config.Check"], "error in"=w321) -> ("error out"=w320:errorcluster)  [unwired: 10 in, 2 out]
              }
              event "Number of Cycles": Value Change {
                n153 = event-data() -> ()  [unwired: 1 in, 2 out]
                n154 = call <vilib>:"Send Local Messages.vi"("message queue in"=w324, "message names"=string[] ["Config.Check", "UI.UpdateTotalIterations"], "error in"=w326) -> ("error out"=w325:errorcluster)  [unwired: 10 in, 2 out]
              }
              event "View": Value Change {
                n155 = event-data() -> ("NewVal"=w331:enum16{"Graph", "Table"})  [unwired: 1 in]
                n156 = case shown="\"Graph\"" w331 {
                  tunnel: [TRUE FALSE] -> w330
                  frame "Graph" {
                  }
                  frame "Table" {
                  }
                }
                n157 = Unbundle By Name(w337) -> ("UI.Table"=w335:refnum<vi>, "UI.Chart"=w336:refnum<vi>)
                n158 = property class="WFChart (strict)"(reference=w336, error in=w333, "Visible"=w330) -> (error out=w334:errorcluster)  [unwired: 1 out]
                n159 = Not(x=w330) -> (.not. x?=w329:bool)
                n160 = property class="MCListbox (strict)"(reference=w335, error in=w334, "Visible"=w329) -> (error out=w332:errorcluster)  [unwired: 1 out]
              }
              event User Event {
                n161 = event-data() -> ("Workspace Event"=w340:string)  [unwired: 1 in]
                n162 = Unbundle By Name(w345) -> ("NIVS.SequenceState"=w344:T4)
                n163 = Equal?(x="Shut Down" ("y"), y=w340) -> (x = y?=w346:bool)
                n164 = case shown="True" w346 {
                  tunnel: w344 -> [_ _]
                  tunnel: w343 -> [w348 w353]
                  tunnel: [w348 w352] -> w342
                  tunnel: w341 -> [_ w351]
                  frame False {
                  }
                  frame True {
                    n165 = Build Array("Macro.Exit" ("y")) -> (w350:string[])
                    n166 = call <vilib>:"Send Local Messages.vi"("message queue in"=w351, "message names"=w350, "error in"=w353) -> ("error out"=w352:errorcluster)  [unwired: 10 in, 2 out]
                  }
                }
              }
            }
          }
          frame "Acq.Start" {
            n167 = Unbundle By Name(w361) -> ("UDP.Queue"=w360:refnum<queue>, "Sequence.Channels"=w356:string[], "INI.Settings.PlotChannels"=w357:string[])
            n168 = Build Array (concatenate)(w356, w357) -> (w355:string[])
            n169 = Empty Array?(array=w355) -> (empty?=w354:bool)
            n170 = case shown="False" w354 {
              tunnel: w360 -> [w367 _]
              tunnel: w359 -> [w364 w368]
              tunnel: [w363 w368] -> w358
              tunnel: w355 -> [w362 _]
              frame False {
                n171 = Bundle By Name(cluster=T2 {"Action"=enum."Start Acq", "Channels"=[]} ("element"), "Channels"=w362) -> (w365:T2)
                n172 = Enqueue Element(queue=w367, element=w365, error in (no error)=w364) -> (error out=w363:errorcluster)  [unwired: 1 in, 2 out]
              }
              frame True {
              }
            }
          }
          frame "Acq.Stop" {
            n173 = Unbundle By Name(w373) -> ("UDP.Queue"=w372:refnum<queue>)
            n174 = Enqueue Element(queue=w372, element=T2 {"Action"=enum."Stop Acq", "Channels"=[]}, error in (no error)=w371) -> (error out=w370:errorcluster)  [unwired: 1 in, 2 out]
          }
          frame "Acq.Exit" {
            n175 = Unbundle By Name(w378) -> ("UDP.Queue"=w377:refnum<queue>)
            n176 = Enqueue Element(queue=w377, element=T2 {"Action"=enum."Exit", "Channels"=[]}, error in (no error)=w376) -> (error out=w375:errorcluster)  [unwired: 1 in, 2 out]
          }
          frame "Alarms.Get" {
            n177 = call "Alarms.Get.vi"("error in (no error)"=w384, "Cluster"=w383) -> ("error out"=w380:errorcluster)  [unwired: 9 in]
            n178 = call <vilib>:"Send Local Message.vi"("message queue in"=w381, "message name"="Alarms.Select", "error in"=w380) -> ("error out"=w379:errorcluster)  [unwired: 10 in, 2 out]
          }
          frame "Alarms.Select" {
            n179 = call "Alarms.Select.vi"("error in (no error)"=w385, "Cluster"=w386) -> ("error out"=w387:errorcluster)  [unwired: 9 in]
          }
          frame "Alarms.Set" {
            n180 = call "Alarms.Set.vi"("error in (no error)"=w392, "Cluster"=w393) -> ("error out"=w390:errorcluster)  [unwired: 9 in]
            n181 = call <vilib>:"Send Local Message.vi"("message queue in"=w388, "message name"="Alarms.Select", "error in"=w390) -> ("error out"=w389:errorcluster)  [unwired: 10 in, 2 out]
          }
          frame "Alarms.TempChange" {
            w399 = T15."Enabled" ("Disabled")
            n182 = Unbundle By Name(w398) -> ("UI.Apply"=w395:refnum<vi>, "UI.Revert"=w394:refnum<vi>)
            n183 = property class="Bool"(reference=w394, error in=w397, "DisabledEnum"=w399) -> (error out=w400:errorcluster)  [unwired: 1 out]
            n184 = property class="Bool"(reference=w395, error in=w400, "DisabledEnum"=w399) -> (error out=w396:errorcluster)  [unwired: 1 out]
          }
          frame "Alarms.DisableAll" {
            n185 = call "Alarms.DisableALl.vi"("error in (no error)"=w403, "Cluster"=w401) -> ("error out"=w402:errorcluster)  [unwired: 9 in]
          }
          frame "App.CloseReferences" {
            n186 = flat-sequence {
              tunnel: [w414] -> w404
              tunnel: w405 -> [w414]
              tunnel: [w413] -> _
              frame #0 {
                n187 = invoke class="VI" method="FP.Close"() -> (error out=w413:errorcluster)  [unwired: 3 in, 2 out]
                n188 = Wait (ms)(milliseconds to wait=u32 500) -> ()  [unwired: 1 out]
              }
            }
            n189 = Unbundle By Name(w404) -> ("Events.State"=w409:refnum<user-event>, "Events.Test Result"=w410:refnum<user-event>, "Events.Progress"=w411:refnum<user-event>, "NIVS.Events"=w406:T10, "NIVS.SystemStateRefs"=w408:T12, "NIVS.WorkspaceManager"=w407:T13)
            n190 = call <vilib>:"NI VeriStand - Close Workspace Manager Reference.vi"("WorkspaceManager"=w407) -> ()  [unwired: 10 in, 1 out]
            n191 = call <vilib>:"NI VeriStand - Close Engine State Change Notification.vi"("SystemStateRefs"=w408) -> ()  [unwired: 10 in, 1 out]
            n192 = Unregister For Events(event registration refnum=w406) -> ()  [unwired: 1 in, 1 out]
            n193 = Destroy User Event(user event=w411) -> ()  [unwired: 1 in, 1 out]
            n194 = Destroy User Event(user event=w410) -> ()  [unwired: 1 in, 1 out]
            n195 = Destroy User Event(user event=w409) -> ()  [unwired: 1 in, 1 out]
          }
          frame "App.CreateEvents" {
            n196 = call "Execute.CreateEvents.vi"("error in (no error)"=w417, "Cluster in"=w416) -> ("error out"=w419:errorcluster, "Cluster out"=w418:T5)  [unwired: 8 in]
          }
          frame "App.CreateFolders" {
            n197 = Unbundle By Name(w429) -> ("NIVS.BaseToolPath"=w422:path, "NIVS.BaseLogPath"=w428:path)
            n198 = Build Path(base path=w422, name or relative path="Configurations") -> (appended path=w421:path)
            n199 = flat-sequence {
              tunnel: w428 -> [w433]
              tunnel: w426 -> [w432]
              tunnel: [w432] -> w425
              tunnel: [w431] -> w424
              tunnel: w421 -> [w430]
              tunnel: [w430] -> w420
              tunnel: [w436] -> _
              tunnel: [w437] -> w427
              tunnel: w425 -> [w437]
              tunnel: w424 -> [w436]
              tunnel: w420 -> [w435]
              tunnel: [w434] -> _
              frame #0 {
                n200 = Create Folder(path (use dialog)=w433) -> (error out=w431:errorcluster)  [unwired: 2 in, 2 out]
              }
              frame #1 {
                n201 = Create Folder(path (use dialog)=w435) -> (error out=w434:errorcluster)  [unwired: 2 in, 2 out]
              }
            }
          }
          frame "App.Exit" {
            n202 = call <vilib>:"Destroy Message Queue.vi"("message queue in"=w443, "error in"=w442) -> ("error out"=w441:errorcluster)  [unwired: 11 in, 2 out]
            n203 = Unbundle By Name(w440) -> ("UI.Multihead"=w439:refnum<vi>)
            n204 = property class="Bool (strict)"(reference=w439, "Value"=FALSE) -> ()  [unwired: 1 in, 2 out]
          }
          frame "App.Initialize" {
            n205 = call "Execute.Initialize.vi"("error in (no error)"=w454, "Cluster"=w449) -> ("error out"=w447:errorcluster)  [unwired: 9 in]
            n206 = call "Tool.GetPath.vi"("error in (no error)"=w447, "Cluster"=w449) -> ("error out"=w446:errorcluster, "path"=w445:path)  [unwired: 8 in]
            n207 = call "INI.GetSettings.vi"("error in (no error)"=w446, "INI Folder Location"=w445, "State Variables"=w449) -> ("error out"=w453:errorcluster, "INI.Settings"=w451:T6)  [unwired: 7 in]
            n208 = Bundle By Name(cluster=w449, "NIVS.BaseToolPath"=w445, "Sequence.Channels"=string[] [], "Restart.Path"=path "", "INI.Settings"=w451) -> (w452:T5)
          }
          frame "App.New" {
            n209 = call <vilib>:"Send Local Message.vi"("message queue in"=w458, "message name"="Macro.New", "error in"=w457) -> ("error out"=w456:errorcluster)  [unwired: 10 in, 2 out]
          }
          frame "App.Restart" {
            n210 = Unbundle By Name(w465) -> ("NIVS.BaseLogPath"=w464:path)
            n211 = call "File Dialog"("start path"=w464, "prompt"="Select the restart file.", "button label"="Select", "error in"=w470, "pattern (all files)"="*.info", "pattern label"="Restart Info") -> ("selected path"=w467:path, "cancelled"=w471:bool, "error out"=w468:errorcluster)  [unwired: 6 in, 1 out]
            n212 = case shown="False" w471 {
              tunnel: w465 -> [w478 w489]
              tunnel: [w480 w489] -> w472
              tunnel: [w474 w487] -> w469
              tunnel: w468 -> [w479 w488]
              tunnel: w467 -> [w477 _]
              tunnel: w460 -> [w473 _]
              frame False {
                n213 = call "Restart.CheckValidSelection.vi"("error in (no error)"=w479, "Restart Path"=w477, "State Variables"=w478) -> ("error out"=w475:errorcluster, "Load Restart?"=w476:bool, "State Variables out"=w480:T5)  [unwired: 6 in]
                n214 = case shown="True" w476 {
                  tunnel: w475 -> [w481 w485]
                  tunnel: [w481 w483] -> w474
                  tunnel: w473 -> [_ w482]
                  frame False {
                  }
                  frame True {
                    n215 = Build Array("UI.StimulusRestart") -> (w484:string[])
                    n216 = call <vilib>:"Send Local Messages.vi"("message queue in"=w482, "message names"=w484, "error in"=w485) -> ("error out"=w483:errorcluster)  [unwired: 10 in, 2 out]
                  }
                }
              }
              frame True {
                n217 = call <vilib>:"Clear Errors.vi"("error in (no error)"=w488) -> ("error out"=w487:errorcluster)  [unwired: 5 in, 1 out]
              }
            }
          }
          frame "Config.Check" {
            n218 = call "Config.Check.vi"("error in (no error)"=w500, "State Variables"=w492) -> ("error out"=w499:errorcluster, "Valid Config?"=w490:bool)  [unwired: 8 in]
            n219 = Bundle By Name(cluster=w492, "Sequence.ValidConfig?"=w490) -> (w491:T5)
            n220 = Select(t="Configuration is Valid.  Ready to Run..." ("message name"), s=w490, f="Configuration is Invalid..." ("message name")) -> (s? t:f=w493:string)
            n221 = call <vilib>:"Send Local Message.vi"("message queue in"=w497, "message name"="UI.UpdateStatus", "message value"=w493, "error in"=w499) -> ("error out"=w498:errorcluster)  [unwired: 9 in, 2 out]
          }
          frame "Config.Load" {
            n222 = Unbundle By Name(w505) -> ("NIVS.BaseToolPath"=w502:path)
            n223 = Build Path(base path=w502, name or relative path="Configurations") -> (appended path=w501:path)
            n224 = call "File Dialog3"("start path"=w501, "prompt"="Load the configuration file.", "button label"="Load", "error in"=w510, "pattern (all files)"="*.dat", "pattern label"="Configuration") -> ("selected path"=w506:path, "cancelled"=w509:bool, "error out"=w508:errorcluster)  [unwired: 6 in, 1 out]
            n225 = case shown="False" w509 {
              tunnel: w508 -> [w521 w523]
              tunnel: [w517 w522] -> w507
              tunnel: w505 -> [w520 _]
              tunnel: w506 -> [w519 _]
              tunnel: w504 -> [w516 _]
              frame False {
                n226 = call "Config.Load.vi"("error in (no error)"=w521, "Cluster"=w520, "selected path"=w519) -> ("error out"=w518:errorcluster)  [unwired: 8 in]
                n227 = call <vilib>:"Send Local Messages.vi"("message queue in"=w516, "message names"=string[] ["Config.Check", "Alarms.Select"], "error in"=w518) -> ("error out"=w517:errorcluster)  [unwired: 10 in, 2 out]
              }
              frame True {
                n228 = call <vilib>:"Clear Errors.vi"("error in (no error)"=w523) -> ("error out"=w522:errorcluster)  [unwired: 5 in, 1 out]
              }
            }
          }
          frame "Config.Save" {
            n229 = Unbundle By Name(w525) -> ("NIVS.BaseToolPath"=w526:path)
            n230 = Build Path(base path=w526, name or relative path="Configurations") -> (appended path=w524:path)
            n231 = call "File Dialog2"("start path"=w524, "prompt"="Save the configuration file.", "button label"="Save", "error in"=w532, "pattern (all files)"="*.dat", "pattern label"="Configuration") -> ("selected path"=w528:path, "cancelled"=w531:bool, "error out"=w530:errorcluster)  [unwired: 6 in, 1 out]
            n232 = case shown="False" w531 {
              tunnel: w530 -> [w540 w542]
              tunnel: [w537 w541] -> w529
              tunnel: w525 -> [w538 _]
              tunnel: w528 -> [w539 _]
              frame False {
                n233 = call "Config.Save.vi"("error in (no error)"=w540, "Cluster"=w538, "selected path"=w539) -> ("error out"=w537:errorcluster)  [unwired: 8 in]
              }
              frame True {
                n234 = call <vilib>:"Clear Errors.vi"("error in (no error)"=w542) -> ("error out"=w541:errorcluster)  [unwired: 5 in, 1 out]
              }
            }
          }
          frame "Error" {
            n235 = Unbundle By Name(w544) -> ("NIVS.SequenceState"=w543:T4)
            n236 = for {
              shift-right: [w560] -> w546
              shift-left: w548 -> [w561]
              tunnel: i32[] [-307652, -307654] -> [w559] mode=indexing
              n237 = call <vilib>:"Clear Errors.vi"("error in (no error)"=w561, "specific error code to clear (0: all)"=w559) -> ("error out"=w560:errorcluster)  [unwired: 4 in, 1 out]
            }
            n238 = case shown="Error" w546 {
              selector: w546 -> [w550 w551]
              tunnel: [w550 w555] -> w549
              tunnel: w545 -> [_ w553]
              tunnel: w543 -> [_ w552]
              frame No Error {
              }
              frame Error {
                n239 = case shown="Default" w552 {
                  tunnel: [string[] ["Stimulus.Stop"] string[] ["UI.SetBusy", "Stimulus.Stop", "Stimulus.Close", "Stimulus.UnregisterCallbacks", "Acq.Stop", "App.Initialize", "NIVS.CheckDeployment", "Page.Publish", "UI.StimulusComplete", "UI.UnsetBusy"]] -> w554
                  frame Default {
                  }
                  frame "Idle" {
                  }
                }
                n240 = call "Error.Display.vi"("error in (no error)"=w551) -> ()  [unwired: 11 in]
                n241 = call <vilib>:"Clear Errors.vi"("error in (no error)"=w551) -> ("error out"=w556:errorcluster)  [unwired: 5 in, 1 out]
                n242 = call <vilib>:"Send Local Messages.vi"("message queue in"=w553, "message names"=w554, "error in"=w556) -> ("error out"=w555:errorcluster)  [unwired: 10 in, 2 out]
              }
            }
          }
          frame "INI.Open" {
            n243 = Unbundle By Name(w569) -> ("NIVS.BaseToolPath"=w562:path)
            n244 = global read "Main.Constants.vi" "INI.FileName"() -> (w570:string)
            n245 = Build Path(base path=w562, name or relative path=w570) -> (appended path=w566:path)
            n246 = Path To String(path=w566) -> (string=w565:string)
            n247 = Concatenate Strings("explorer " ("string"), w565) -> (w563:string)
            n248 = call <vilib>:"System Exec.vi"("error in (no error)"=w568, "command line"=w563) -> ("error out"=w567:errorcluster)  [unwired: 6 in, 3 out]
          }
          frame "Macro.Exit" {
            n249 = Unbundle By Name(w574) -> ("NIVS.SequenceState"=w575:T4)
            n250 = case shown="\"Idle\", \"Complete\"" w575 {
              tunnel: w573 -> [w577 w583]
              tunnel: [w576 w582] -> w572
              tunnel: w571 -> [w578 w581]
              frame "Idle", "Complete" {
                n251 = call <vilib>:"Send Local Messages.vi"("message queue in"=w578, "message names"=string[] ["Stimulus.Stop", "Stimulus.Close", "Stimulus.UnregisterCallbacks", "Acq.Stop", "Acq.Exit", "App.CloseReferences", "App.Exit"], "error in"=w577) -> ("error out"=w576:errorcluster)  [unwired: 10 in, 2 out]
              }
              frame Default {
                n252 = call <vilib>:"Send Local Messages.vi"("message queue in"=w581, "message names"=string[] ["Stimulus.Stop", "Stimulus.Close", "Stimulus.CacheRestart", "Stimulus.UnregisterCallbacks", "Acq.Stop", "Acq.Exit", "App.CloseReferences", "App.Exit"], "error in"=w583) -> ("error out"=w582:errorcluster)  [unwired: 10 in, 2 out]
              }
            }
          }
          frame "Macro.Run" {
            n253 = call <vilib>:"Send Local Messages.vi"("message queue in"=w584, "message names"=string[] ["UI.SetBusy", "Stimulus.Close", "Stimulus.UnregisterCallbacks", "Stimulus.Create", "Stimulus.RegisterCallbacks", "Acq.Start", "Stimulus.Run", "UI.StimulusRunning", "UI.UnsetBusy"] ("array"), "error in"=w586) -> ("error out"=w585:errorcluster)  [unwired: 10 in, 2 out]
          }
          frame "Macro.New" {
            n254 = call <vilib>:"Send Local Messages.vi"("message queue in"=w591, "message names"=string[] ["UI.SetBusy", "App.Initialize", "NIVS.CheckDeployment", "Page.Publish", "UI.UnsetBusy"], "error in"=w590) -> ("error out"=w589:errorcluster)  [unwired: 10 in, 2 out]
          }
          frame "Macro.Restart" {
            n255 = call <vilib>:"Send Local Messages.vi"("message queue in"=w596, "message names"=string[] ["UI.SetBusy", "Stimulus.Close", "Stimulus.UnregisterCallbacks", "Stimulus.Open", "Alarms.Select", "Stimulus.RegisterCallbacks", "Acq.Start", "Stimulus.Run", "UI.StimulusRunning", "UI.UnsetBusy"] ("array"), "error in"=w595) -> ("error out"=w594:errorcluster)  [unwired: 10 in, 2 out]
          }
          frame "NIVS.CheckDeployment" {
            n256 = call "NIVS.CheckDeployed.vi"("error in (no error)"=w604, "Cluster in"=w606) -> ("error out"=w603:errorcluster, "System State"=w599:T19, "Cluster out"=w605:T5)  [unwired: 7 in]
            n257 = case shown="1" w599 {
              tunnel: [string[] ["Config.Check", "Alarms.Get", "UI.UpdateStatus"] string[] ["Config.Check", "Alarms.Get", "App.CreateFolders", "UI.UpdateStatus"]] -> w600
              frame 0, Default {
                # "Not connected"
              }
              frame 1 {
                # "Connected"
              }
            }
            n258 = call <vilib>:"Send Local Messages.vi"("message queue in"=w601, "message names"=w600, "error in"=w603) -> ("error out"=w602:errorcluster)  [unwired: 10 in, 2 out]
          }
          frame "Page.Back" {
            n259 = Unbundle By Name(w609) -> ("UI.Next"=w613:refnum<vi>, "UI.Back"=w620:refnum<vi>, "UI.TabControl"=w625:refnum<vi>)
            n260 = property class="TabCtl (strict)"(reference=w625, error in=w610) -> (reference out=w623:refnum<vi>, error out=w622:errorcluster, "Value"=w624:enum32{"Metadata", "Alarms", "Execution"})
            n261 = Decrement(x=w624) -> (x-1=w619:enum32{"Metadata", "Alarms", "Execution"})
            n262 = Equal To 0?(x=w619) -> (x = 0?=w618:bool)
            n263 = property class="TabCtl (strict)"(reference=w623, error in=w622, "Value"=w619) -> (error out=w621:errorcluster)  [unwired: 1 out]
            n264 = Select(t=T15."Disabled and Grayed Out" ("Disabled"), s=w618, f=T15."Enabled") -> (s? t:f=w615:T15)
            n265 = property class="Bool"(reference=w620, error in=w621, "DisabledEnum"=w615) -> (error out=w614:errorcluster)  [unwired: 1 out]
            n266 = property class="Bool"(reference=w613, error in=w614, "DisabledEnum"=T15."Enabled" ("Disabled")) -> (error out=w611:errorcluster)  [unwired: 1 out]
          }
          frame "Page.Next" {
            n267 = Unbundle By Name(w630) -> ("UI.Back"=w646:refnum<vi>, "UI.Next"=w645:refnum<vi>, "UI.TabControl"=w644:refnum<vi>)
            n268 = property class="TabCtl (strict)"(reference=w644, error in=w628) -> (reference out=w632:refnum<vi>, error out=w633:errorcluster, "Value"=w631:enum32{"Metadata", "Alarms", "Execution"}, "Pages"=w627:refnum<vi>[])
            n269 = To Unsigned Byte Integer(number=w631) -> (unsigned 8bit integer=w643:u8)
            n270 = Array Size(array=w627) -> (size(s)=w626:i32)
            n271 = Increment(x=w643) -> (x+1=w634:u8)
            n272 = Increment(x=w634) -> (x+1=w635:u8)
            n273 = property class="TabCtl (strict)"(reference=w632, error in=w633, "Value"=w634) -> (error out=w636:errorcluster)  [unwired: 1 out]
            n274 = Greater Or Equal?(x=w635, y=w626) -> (x >= y?=w641:bool)
            n275 = Select(t=T15."Disabled and Grayed Out" ("Disabled"), s=w641, f=T15."Enabled") -> (s? t:f=w642:T15)
            n276 = property class="Bool"(reference=w645, error in=w636, "DisabledEnum"=w642) -> (error out=w637:errorcluster)  [unwired: 1 out]
            n277 = property class="Bool"(reference=w646, error in=w637, "DisabledEnum"=T15."Enabled" ("Disabled")) -> (error out=w629:errorcluster)  [unwired: 1 out]
          }
          frame "Page.Publish" {
            n278 = Unbundle By Name(w661) -> ("Station.ID"=w655:string, "UI.TabControl"=w660:refnum<vi>)
            n279 = property class="TabCtl (strict)"(reference=w660, error in=w647) -> (error out=w656:errorcluster, "Value"=w658:enum32{"Metadata", "Alarms", "Execution"}, "Pages"=w659:refnum<vi>[])  [unwired: 1 out]
            n280 = Index Array(array=w659, index=w658) -> (element=w657:refnum<vi>)
            n281 = property class="Page"(reference=w657, error in=w656) -> (error out=w651:errorcluster, "PageLabel"=w654:string)  [unwired: 1 out]
            n282 = Concatenate Strings(w655, "\\" ("string"), w654) -> (w652:string)
            n283 = call <vilib>:"Send Local Message.vi"("receiver process (\"\" - local)"="MainExecutionTool" ("string"), "message name"="Page.Published" ("string"), "message value"=w652, "error in"=w651) -> ("error out"=w648:errorcluster)  [unwired: 9 in, 2 out]
            n284 = call <vilib>:"Clear Errors.vi"("error in (no error)"=w648) -> ()  [unwired: 5 in, 2 out]
          }
          frame "Page.Set" {
            n285 = call "Page.Set.vi"("error in (no error)"=w663, "message value"=w664, "Cluster"=w665) -> ("error out"=w662:errorcluster)  [unwired: 8 in]
          }
          frame "Tool.Disable" {
            n286 = Unbundle By Name(w670) -> ("UI.ToolTab"=w669:refnum<vi>)
            n287 = property class="TabCtl (strict)"(reference=w669, error in=w668, "Value"=enum32{"Enable", "Disable"}."Disable") -> (error out=w667:errorcluster)  [unwired: 1 out]
          }
          frame "Tool.Enable" {
            n288 = Unbundle By Name(w675) -> ("UI.ToolTab"=w674:refnum<vi>)
            n289 = property class="TabCtl (strict)"(reference=w674, error in=w673, "Value"=enum32{"Enable", "Disable"}."Enable") -> (error out=w672:errorcluster)  [unwired: 1 out]
          }
          frame "Sequence.Open" {
            n290 = call "Execute.OpenSequence.vi"("error in (no error)"=w678, "State Variables"=w676) -> ("error out"=w677:errorcluster)  [unwired: 9 in]
          }
          frame "Stimulus.CacheRestart" {
            n291 = call "Restart.CacheCurrentLocation.vi"("error in (no error)"=w685, "Result"=Results.Value."Aborted", "State Variables"=w682) -> ("error out"=w684:errorcluster, "State Variables out"=w681:T5)  [unwired: 6 in, 1 out]
            n292 = Bundle By Name(cluster=w681, "Restart.Path"=path "") -> (w680:T5)
          }
          frame "Stimulus.Close" {
            n293 = call "Stimulus.Close.vi"("Cluster"=w687) -> ("output cluster"=w686:T5)  [unwired: 10 in]
          }
          frame "Stimulus.Continue" {
            n294 = Unbundle By Name(w693) -> ("NIVS.SequenceState"=w692:T4, "NIVS.ProfileRef"=w691:refnum<k24>)
            n295 = case shown="\"Paused\"" w692 {
              tunnel: w691 -> [_ w697]
              tunnel: w690 -> [w694 w696]
              tunnel: [w694 w695] -> w689
              frame "Idle", Default {
              }
              frame "Paused" {
                n296 = invoke class="StimulusProfile" method="Continue"(reference=w697, error in=w696) -> (error out=w695:errorcluster)  [unwired: 1 in, 2 out]
              }
            }
          }
          frame "Stimulus.Create" {
            n297 = call "Stimulus.Create.vi"("error in (no error)"=w701, "State Variables"=w699) -> ("error out"=w700:errorcluster, "State Variables"=w698:T5)  [unwired: 8 in]
          }
          frame "Stimulus.GetStatus" {
            n298 = Unbundle By Name(w713) -> ("source process"=w712:string)
            n299 = call "Stimulus.GetStatus.vi"("error in (no error)"=w704, "Cluster"=w709) -> ("error out"=w706:errorcluster, "cluster"=w705:T20)  [unwired: 8 in]
            n300 = Flatten To String(anything=w705, error in (no error)=w706) -> (data string=w708:string, error out=w702:errorcluster)  [unwired: 2 in, 1 out]
            n301 = Concatenate Strings(w707, "Response" ("string")) -> (w710:string)
            n302 = call <vilib>:"Send Local Message.vi"("receiver process (\"\" - local)"=w712, "message name"=w710, "message value"=w708, "error in"=w702) -> ("error out"=w703:errorcluster)  [unwired: 9 in, 2 out]
            n303 = call <vilib>:"Clear Errors.vi"("error in (no error)"=w703) -> ()  [unwired: 5 in, 2 out]
          }
          frame "Stimulus.Open" {
            n304 = call "Stimulus.Open.vi"("error in (no error)"=w717, "State Variables"=w715) -> ("error out"=w716:errorcluster, "State Variables"=w714:T5)  [unwired: 8 in]
          }
          frame "Stimulus.Pause" {
            n305 = Unbundle By Name(w722) -> ("NIVS.SequenceState"=w720:T4, "NIVS.ProfileRef"=w721:refnum<k24>)
            n306 = case shown="\"Running\"" w720 {
              tunnel: w721 -> [_ w726]
              tunnel: w719 -> [w723 w725]
              tunnel: [w723 w724] -> w718
              frame "Idle", Default {
              }
              frame "Running" {
                n307 = invoke class="StimulusProfile" method="Pause"(reference=w726, error in=w725) -> (error out=w724:errorcluster)  [unwired: 1 in, 2 out]
              }
            }
          }
          frame "Stimulus.RegisterCallbacks" {
            n308 = Unbundle By Name(w730) -> ("NIVS.ProfileRef"=w736:refnum<k24>, "Events.Progress"=w735:refnum<user-event>, "Events.Test Result"=w734:refnum<user-event>, "Events.State"=w733:refnum<user-event>)
            n309 = vi-ref "SequenceEvent.ProgressChanged.vi"() -> ("vi reference"=w729:refnum<vi>)
            n310 = vi-ref "SequenceEvent.ExecuteCompleted.vi"() -> ("vi reference"=w728:refnum<vi>)
            n311 = vi-ref "SequenceEvent.PropertyChanged.vi"() -> ("vi reference"=w727:refnum<vi>)
            n312 = node(w738, w736, w729, w735, w736, w728, w734, w736, w727, w733) -> (w732:refnum<k27>, w737:errorcluster)  [unwired: 1 in]
            n313 = Bundle By Name(cluster=w730, "NIVS.ProfileCallback"=w732) -> (w731:T5)
          }
          frame "Stimulus.Run" {
            n314 = call "Stimulus.Run.vi"("error in (no error)"=w742, "Cluster in"=w741) -> ("error out"=w739:errorcluster, "Cluster out"=w740:T5)  [unwired: 8 in]
          }
          frame "Stimulus.Stop" {
            n315 = Unbundle By Name(w747) -> ("NIVS.WorkspaceManager"=w743:T13, "INI.Settings.Sequence.AbortChannel"=w744:string, "NIVS.SequenceState"=w745:T4, "NIVS.ProfileRef"=w746:refnum<k24>)
            n316 = case shown="\"Running\", \"Paused\", Default" w745 {
              tunnel: w746 -> [_ w752]
              tunnel: w749 -> [w750 w756]
              tunnel: [w750 w751] -> w748
              tunnel: w744 -> [_ w755]
              tunnel: w743 -> [_ w754]
              frame "Idle" {
              }
              frame "Running", "Paused", Default {
                n317 = case shown="Default" w755 {
                  selector: w755 -> [_ w758]
                  tunnel: w756 -> [w757 w764]
                  tunnel: [w757 w760] -> w753
                  tunnel: w754 -> [_ w763]
                  frame "" {
                  }
                  frame Default {
                    n318 = call-poly <vilib>:"NI VeriStand - Set Channel Value.vi"("error in (no error)"=w764, "Value"=1.0, "Channel"=w758, "WorkspaceManager in"=w763) -> ("error out"=w761:errorcluster)  [unwired: 6 in, 1 out]
                    n319 = flat-sequence {
                      tunnel: w761 -> [w766]
                      tunnel: [w766] -> w760
                      tunnel: 100 -> [w765]
                      frame #0 {
                        n320 = Wait (ms)(milliseconds to wait=w765) -> ()  [unwired: 1 out]
                      }
                    }
                  }
                }
                n321 = invoke class="StimulusProfile" method="Stop"(reference=w752, error in=w753) -> (error out=w751:errorcluster)  [unwired: 1 in, 2 out]
              }
            }
          }
          frame "Stimulus.UnregisterCallbacks" {
            n322 = Unbundle By Name(w768) -> ("NIVS.ProfileCallback"=w767:refnum<k27>)
            n323 = flat-sequence {
              tunnel: w767 -> [w771]
              tunnel: [w770] -> _
              frame #0 {
                n324 = Unregister For Events(event registration refnum=w771) -> (error out=w770:errorcluster)  [unwired: 1 in]
              }
            }
          }
          frame "UI.Open" {
            n325 = invoke class="VI" method="FP.Open"(error in=w773) -> (error out=w772:errorcluster)  [unwired: 4 in, 4 out]
          }
          frame "UI.SetBusy" {
            n326 = call <vilib>:"Send Local Message.vi"("receiver process (\"\" - local)"="MainExecutionTool" ("string"), "message name"=w775, "error in"=w776) -> ("error out"=w777:errorcluster)  [unwired: 10 in, 2 out]
            n327 = call <vilib>:"Clear Errors.vi"("error in (no error)"=w777) -> ()  [unwired: 5 in, 2 out]
            n328 = call <vilib>:"Set Busy.vi"() -> ()  [unwired: 10 in, 2 out]
          }
          frame "UI.StimulusComplete" {
            n329 = call "UI.StimulusComplete.vi"("error in (no error)"=w782, "Cluster"=w780) -> ("error out"=w781:errorcluster)  [unwired: 9 in]
          }
          frame "UI.StimulusRestart" {
            n330 = call "UI.StimulusRestart.vi"("error in (no error)"=w785, "Cluster"=w783) -> ("error out"=w784:errorcluster)  [unwired: 9 in]
          }
          frame "UI.StimulusRunning" {
            n331 = call "Execute.UI.Running.vi"("error in (no error)"=w788, "Cluster"=w786) -> ("error out"=w787:errorcluster)  [unwired: 9 in]
          }
          frame "UI.UnsetBusy" {
            n332 = call <vilib>:"Send Local Message.vi"("receiver process (\"\" - local)"="MainExecutionTool" ("string"), "message name"=w790, "error in"=w789) -> ("error out"=w791:errorcluster)  [unwired: 10 in, 2 out]
            n333 = call <vilib>:"Clear Errors.vi"("error in (no error)"=w791) -> ()  [unwired: 5 in, 2 out]
            n334 = call <vilib>:"Unset Busy.vi"() -> ()  [unwired: 11 in, 1 out]
          }
          frame "UI.UpdateState" {
            n335 = Unbundle By Name(w807) -> ("UI.Start"=w800:refnum<vi>, "UI.Abort"=w801:refnum<vi>, "UI.Pause"=w805:refnum<vi>, "UI.Skip"=w795:refnum<vi>, "NIVS.SequenceState"=w806:T4)
            n336 = case shown="\"Running\"" w806 {
              tunnel: [w808 w810 T15."Disabled and Grayed Out" ("Disabled") w813] -> w794
              tunnel: [T15."Disabled and Grayed Out" ("Disabled") w810 w812 T15."Enabled" ("f")] -> w799
              tunnel: [w808 w810 w812 w813] -> w802
              frame "Running" {
                w808 = T15."Enabled" ("Disabled")
              }
              frame Default {
                w810 = T15."Disabled and Grayed Out" ("Disabled")
              }
              frame "Paused" {
                w812 = T15."Enabled" ("Disabled")
              }
              frame "Idle" {
                w813 = T15."Disabled and Grayed Out" ("Disabled")
              }
            }
            n337 = property class="Bool"(reference=w795, error in=w797, "DisabledEnum"=w794) -> (error out=w796:errorcluster)  [unwired: 1 out]
            n338 = property class="Bool"(reference=w805, error in=w796, "DisabledEnum"=w794) -> (error out=w804:errorcluster)  [unwired: 1 out]
            n339 = property class="Bool"(reference=w801, error in=w804, "DisabledEnum"=w802) -> (error out=w803:errorcluster)  [unwired: 1 out]
            n340 = property class="Bool"(reference=w800, error in=w803, "DisabledEnum"=w799) -> (error out=w798:errorcluster)  [unwired: 1 out]
          }
          frame "UI.UpdatePreview" {
            n341 = call "UI.UpdatePreview.vi"("error in (no error)"=w815, "Cluster"=w817) -> ("error out"=w816:errorcluster)  [unwired: 9 in]
          }
          frame "UI.UpdateStatus" {
            n342 = Unbundle By Name(w827) -> ("UI.Status"=w824:refnum<vi>, "NIVS.SequenceState"=w825:T4, "NIVS.Deployed"=w826:bool, "UI.Start"=w818:refnum<vi>)
            n343 = case shown="True" w826 {
              tunnel: w825 -> [_ w835]
              tunnel: ["Project Not Deployed.  Please Run VeriStand Project..." w834] -> w822
              tunnel: w821 -> [_ w833]
              tunnel: w820 -> [w828 w832]
              tunnel: [w828 w831] -> w819
              tunnel: w818 -> [_ w830]
              frame False {
              }
              frame True {
                n344 = case shown="\"Idle\"" w835 {
                  selector: w835 -> [_ w844]
                  tunnel: [w837 w839] -> w834
                  tunnel: w833 -> [w837 _]
                  tunnel: w832 -> [w836 w843]
                  tunnel: [w836 w838] -> w831
                  tunnel: w830 -> [_ _]
                  frame "Idle" {
                  }
                  frame Default {
                    n345 = call <userlib>:"Get Strings from Enum__ogtk.vi"("error in (no error)"=w843, "Enum"=w844) -> ("error out"=w838:errorcluster, "String Value"=w841:string)  [unwired: 6 in, 2 out]
                    n346 = Concatenate Strings("Test is ", w841, "..." ("string")) -> (w839:string)
                  }
                }
              }
            }
            n347 = property class="Str"(reference=w824, error in=w819, "Value"=w822) -> (error out=w823:errorcluster)  [unwired: 1 out]
          }
          frame "UI.ClearResults" {
            n348 = Unbundle By Name(w855) -> ("UI.Result"=w847:refnum<vi>, "UI.Log Path"=w852:refnum<vi>, "UI.ReportPath"=w853:refnum<vi>, "UI.RestartPath"=w854:refnum<vi>, "UI.AlarmLog"=w845:refnum<vi>)
            n349 = Build Array(w852, w853, w854, w845) -> (w851:refnum<vi>[])
            n350 = for {
              tunnel: w851 -> [w859] mode=indexing
              shift-right: [w857] -> w849
              shift-left: w850 -> [w858]
              n351 = property class="Path"(reference=w859, error in=w858, "Value"=path "") -> (error out=w857:errorcluster)  [unwired: 1 out]
            }
            n352 = property class="Str"(reference=w847, error in=w849, "Value"="") -> (error out=w848:errorcluster)  [unwired: 1 out]
          }
          frame "UI.UpdateTotalIterations" {
            n353 = Unbundle By Name(w866) -> ("UI.TotalIterations"=w864:refnum<vi>, "UI.NumberOfCycles"=w865:refnum<vi>)
            n354 = property class="DigNum (strict)"(reference=w865, error in=w861) -> (error out=w862:errorcluster, "Value"=w863:u32)  [unwired: 1 out]
            n355 = property class="DigNum (strict)"(reference=w864, error in=w862, "Value"=w863) -> (error out=w860:errorcluster)  [unwired: 1 out]
          }
          frame "UI.UpdateAlarmLog" {
            n356 = Unbundle By Name(w874) -> ("NIVS.SystemDefinitionFile"=w873:path, "UI.AlarmLog"=w868:refnum<vi>)
            n357 = Strip Path(path=w873) -> (stripped path=w872:path)  [unwired: 1 out]
            n358 = Build Path(base path=w872, name or relative path=path "Logs/Alarm Log.txt" ("stripped path")) -> (appended path=w867:path)
            n359 = property class="Path"(reference=w868, error in=w870, "Value"=w867) -> (error out=w869:errorcluster)  [unwired: 1 out]
          }
          frame Default {
          }
        }
      }
      n360 = Unbundle By Name(w70) -> ("UI.Chart"=w68:refnum<vi>, "NIVS.WorkspaceManager"=w67:T13, "UDP.Queue"=w69:refnum<queue>)
      n361 = while {
        tunnel: w69 -> [w79]
        tunnel: w68 -> [w78]
        tunnel: w67 -> [w77]
        tunnel: w66 -> [w73]
        tunnel: w65 -> [w72]
        stop <- w74 stop-if-true
        n362 = call "UDPEngine.Main.vi"("WaveformChart Ref"=w78, "error in (no error)"=w73, "ClientPort"=w72, "UDP Engine Queue"=w79, "WorkspaceManager"=w77) -> ("Exit"=w74:bool, "Update?"=w76:bool, "Waveform"=w75:waveform(dbl)[])  [unwired: 3 in, 1 out]
        n363 = case shown="True" w76 {
          tunnel: w75 -> [_ w80]
          frame False {
          }
          frame True {
            "Chart" <- w80
          }
        }
      }
    }
    frame Error {
      n364 = One Button Dialog(message="NI VeriStand is not open. Please open NI VeriStand before running this utility.") -> (true=w877:bool)  [unwired: 1 in]
      n365 = flat-sequence {
        tunnel: w877 -> [_]
        frame #0 {
          n366 = disable-structure shown="Enabled" {
            frame Enabled {
              n367 = invoke class="VI" method="FP.Close"() -> ()  [unwired: 3 in, 3 out]
            }
            frame Disabled {
            }
          }
        }
      }
    }
  }
  "Station ID" <- "Station.ID"
